vi "MFLMonitor.vi"(0 "Lock-in Reference":u16(ring) items=["Lock-in 1", "Lock-in 2", "Lock-in 3"]) -> ()   [LabVIEW 2019]
uses:
  Utility/Monitor Communication/zurich_lock_in/MFLIMonitor_Cluster.ctl
  Equipment/Zurich Instruments LabOne/Public/Data/ziTypeDemodSampleEx.ctl
  Utility/Monitor Communication/zurich_lock_in/MFLIMonitor-Settings-Cluster.ctl
  Global/Global Variables/Data_Display_global.vi
  Instrument_Setup.vi
  Equipment/Zurich Instruments LabOne/Public/Configure/ziGetValueDouble.vi
  Equipment/Zurich Instruments LabOne/Public/Data/ziGetEventDoubleDataTS.vi
  Equipment/Zurich Instruments LabOne/Public/Data/ziGetEventIntDataTS.vi
  Equipment/Zurich Instruments LabOne/Public/Data/ziGetEventDemodSample.vi
  Equipment/Zurich Instruments LabOne/Public/Configure/ziSetValueDouble.vi
  Equipment/Zurich Instruments LabOne/Zurich Instruments LabOne.lvlib
panel:
  out "Value in Queue":bool
  out "MFLI-1-Settings":T1={"Adress"="DEV4756", "Osc 0 Freq"=0.0, "Osc 1 Freq"=0.0, "Osc 2 Freq"=0.0, "Osc 3 Freq"=0.0, "Demod 0 Osc"=0, "Demod 0 Harm"=1, "Demod 0 Phase"=0.0, "Demod 1 Osc"=0, "Demod 2 Osc"=0, "Demod 3 Osc"=0, "Demod 1 Harm"=1, "Demod 2 Harm"=1, "Demod 3 Harm"=1, "Demod 1 Phase"=0.0, "Demod 2 Phase"=0.0, "Demod 3 Phase"=0.0, "Input Demod 0"="", "Input Demod 1"="", "Input Demod 2"="", "Input Demod 3"="", "Demod 0 Order"=1, "Demod 0 TC"=0.0, "Demod 0 Sinc"=FALSE, "Demod 1 Order"=1, "Demod 2 Order"=1, "Demod 3 Order"=1, "Demod 1 TC"=0.0, "Demod 2 TC"=0.0, "Demod 3 TC"=0.0, "Demod 1 Sinc"=FALSE, "Demod 2 Sinc"=FALSE, "Demod 3 Sinc"=FALSE, "Demod 0 Enable"=FALSE, "Demod 0 Data Rate"=0.0, "Demod 1 Enable"=FALSE, "Demod 2 Enable"=FALSE, "Demod 3 Enable"=FALSE, "Demod 1 Data Rate"=0.0, "Demod 2 Data Rate"=0.0, "Demod 3 Data Rate"=0.0, "Ampl 0"=0.0, "Ampl 0 Enable"=FALSE, "Ampl 1"=0.0, "Ampl 2"=0.0, "Ampl 3"=0.0, "Ampl 1 Enable"=FALSE, "Ampl 2 Enable"=FALSE, "Ampl 3 Enable"=FALSE, "On"=FALSE, "50 Ohm"=FALSE, "Range (V)"=0.0, "Add"=FALSE, "Diff"=FALSE, "Auto-Range"=FALSE, "Offset (V)"=0.0, "Aux Out 0 Select"="", "Aux Out 0 Demod Num"=0.0, "Aux Out 0 Pre Offset"=0.0, "Aux Out 0 Scale"=0.0, "Aux Out 0 Offset"=0.0, "Aux Out 1 Select"="", "Aux Out 2 Select"="", "Aux Out 3 Select"="", "Aux Out 1 Pre Offset"=0.0, "Aux Out 2 Pre Offset"=0.0, "Aux Out 3 Pre Offset"=0.0, "Aux Out 1 Scale"=0.0, "Aux Out 2 Scale"=0.0, "Aux Out 3 Scale"=0.0, "Aux Out 1 Offset"=0.0, "Aux Out 2 Offset"=0.0, "Aux Out 3 Offset"=0.0, "Aux Out 1 Demod Num"=0.0, "Aux Out 2 Demod Num "=0.0, "Aux Out 3 Demod Num"=0.0} {"Aux Out 3 Demod Num" min=0.0 max=3.0 step=1.0; "Aux Out 2 Demod Num" min=0.0 max=3.0 step=1.0; "Aux Out 1 Demod Num" min=0.0 max=3.0 step=1.0; "Aux Out 0 Demod Num" min=0.0 max=3.0 step=1.0; "Demod 3 TC" min=0.0; "Demod 2 TC" min=0.0; "Demod 1 TC" min=0.0; "Demod 3 Order" min=1 max=8 step=1; "Demod 2 Order" min=1 max=8 step=1; "Demod 1 Order" min=1 max=8 step=1; "Demod 0 TC" min=0.0; "Demod 0 Order" min=1 max=8 step=1; "Demod 3 Phase" min=0.0 max=360.0; "Demod 2 Phase" min=0.0 max=360.0; "Demod 1 Phase" min=0.0 max=360.0; "Demod 3 Harm" min=1 max=1023 step=1; "Demod 2 Harm" min=1 max=1023 step=1; "Demod 1 Harm" min=1 max=1023 step=1; "Demod 3 Osc" min=0 max=3 step=1; "Demod 2 Osc" min=0 max=3 step=1; "Demod 1 Osc" min=0 max=3 step=1; "Demod 0 Phase" min=0.0 max=360.0; "Demod 0 Harm" min=1 max=1023 step=1; "Demod 0 Osc" min=0 max=3 step=1; "Osc 3 Freq" min=0.0 max=510000.0 format="%#_11g"; "Osc 2 Freq" min=0.0 max=510000.0 format="%#_11g"; "Osc 1 Freq" min=0.0 max=510000.0 format="%#_11g"; "Osc 0 Freq" min=0.0 max=510000.0 format="%#_11g"}
  in  "Stop":bool
  in  "MFL_Monitor":T2 {"Osc 3 Freq" min=0.0 max=510000.0 format="%#_11g"; "Osc 2 Freq" min=0.0 max=510000.0 format="%#_11g"; "Osc 1 Freq" min=0.0 max=510000.0 format="%#_11g"; "Osc 0 Freq" min=0.0 max=510000.0 format="%#_11g"; "Demod Sample out 3"."Aux In 1 (V)" format="%#_5p"; "Demod Sample out 3"."Aux In 0 (V)" format="%#_5p"; "Demod Sample out 3"."X (Vrms)" format="%#_5p"; "Demod Sample out 3"."Y (Vrms)" format="%#_5p"; "Demod Sample out 3"."Osc Phase (rad)" format="%#.3g"; "Demod Sample out 2"."Aux In 1 (V)" format="%#_5p"; "Demod Sample out 2"."Aux In 0 (V)" format="%#_5p"; "Demod Sample out 2"."X (Vrms)" format="%#_5p"; "Demod Sample out 2"."Y (Vrms)" format="%#_5p"; "Demod Sample out 2"."Osc Phase (rad)" format="%#.3g"; "Demod Sample out 1"."Aux In 1 (V)" format="%#_5p"; "Demod Sample out 1"."Aux In 0 (V)" format="%#_5p"; "Demod Sample out 1"."X (Vrms)" format="%#_5p"; "Demod Sample out 1"."Y (Vrms)" format="%#_5p"; "Demod Sample out 1"."Osc Phase (rad)" format="%#.3g"; "Demod Sample out 0"."Aux In 1 (V)" format="%#_5p"; "Demod Sample out 0"."Aux In 0 (V)" format="%#_5p"; "Demod Sample out 0"."X (Vrms)" format="%#_5p"; "Demod Sample out 0"."Y (Vrms)" format="%#_5p"; "Demod Sample out 0"."Osc Phase (rad)" format="%#.3g"}
  # "Oscillators"
  # "Demodulators"
  # "Low-Pass Filter"
  # "Data Transfer"
  # "Output Amplitudes"
  # "Signal Outputs"
  # "Frequency (Hz)"
  # "Osc (#)"
  # "Harm (#)"
  # "Phase Offset (°)"
  # "Input"
  # "Order (#)"
  # "TC (s)"
  # "Sinc"
  # "Enabled"
  # "Rate (1/s)"
  # "Ampl (Vpk)"
  # "Enable"
  # "0"
  # "0"
  # "0"
  # "1"
  # "1"
  # "1"
  # "2"
  # "2"
  # "2"
  # "3"
  # "3"
  # "3"
  # "Auxiliary Outputs"
  # "Output"
  # "Demod"
  # "Pre Offset"
  # "Scale"
  # "Offset"
  # "0"
  # "1"
  # "2"
  # "3"
  # "Oscillators"
  # "Output Amplitudes"
  # "Frequency (Hz)"
  # "Ampl (Vpk)"
  # "0"
  # "0"
  # "1"
  # "1"
  # "2"
  # "2"
  # "3"
  # "3"
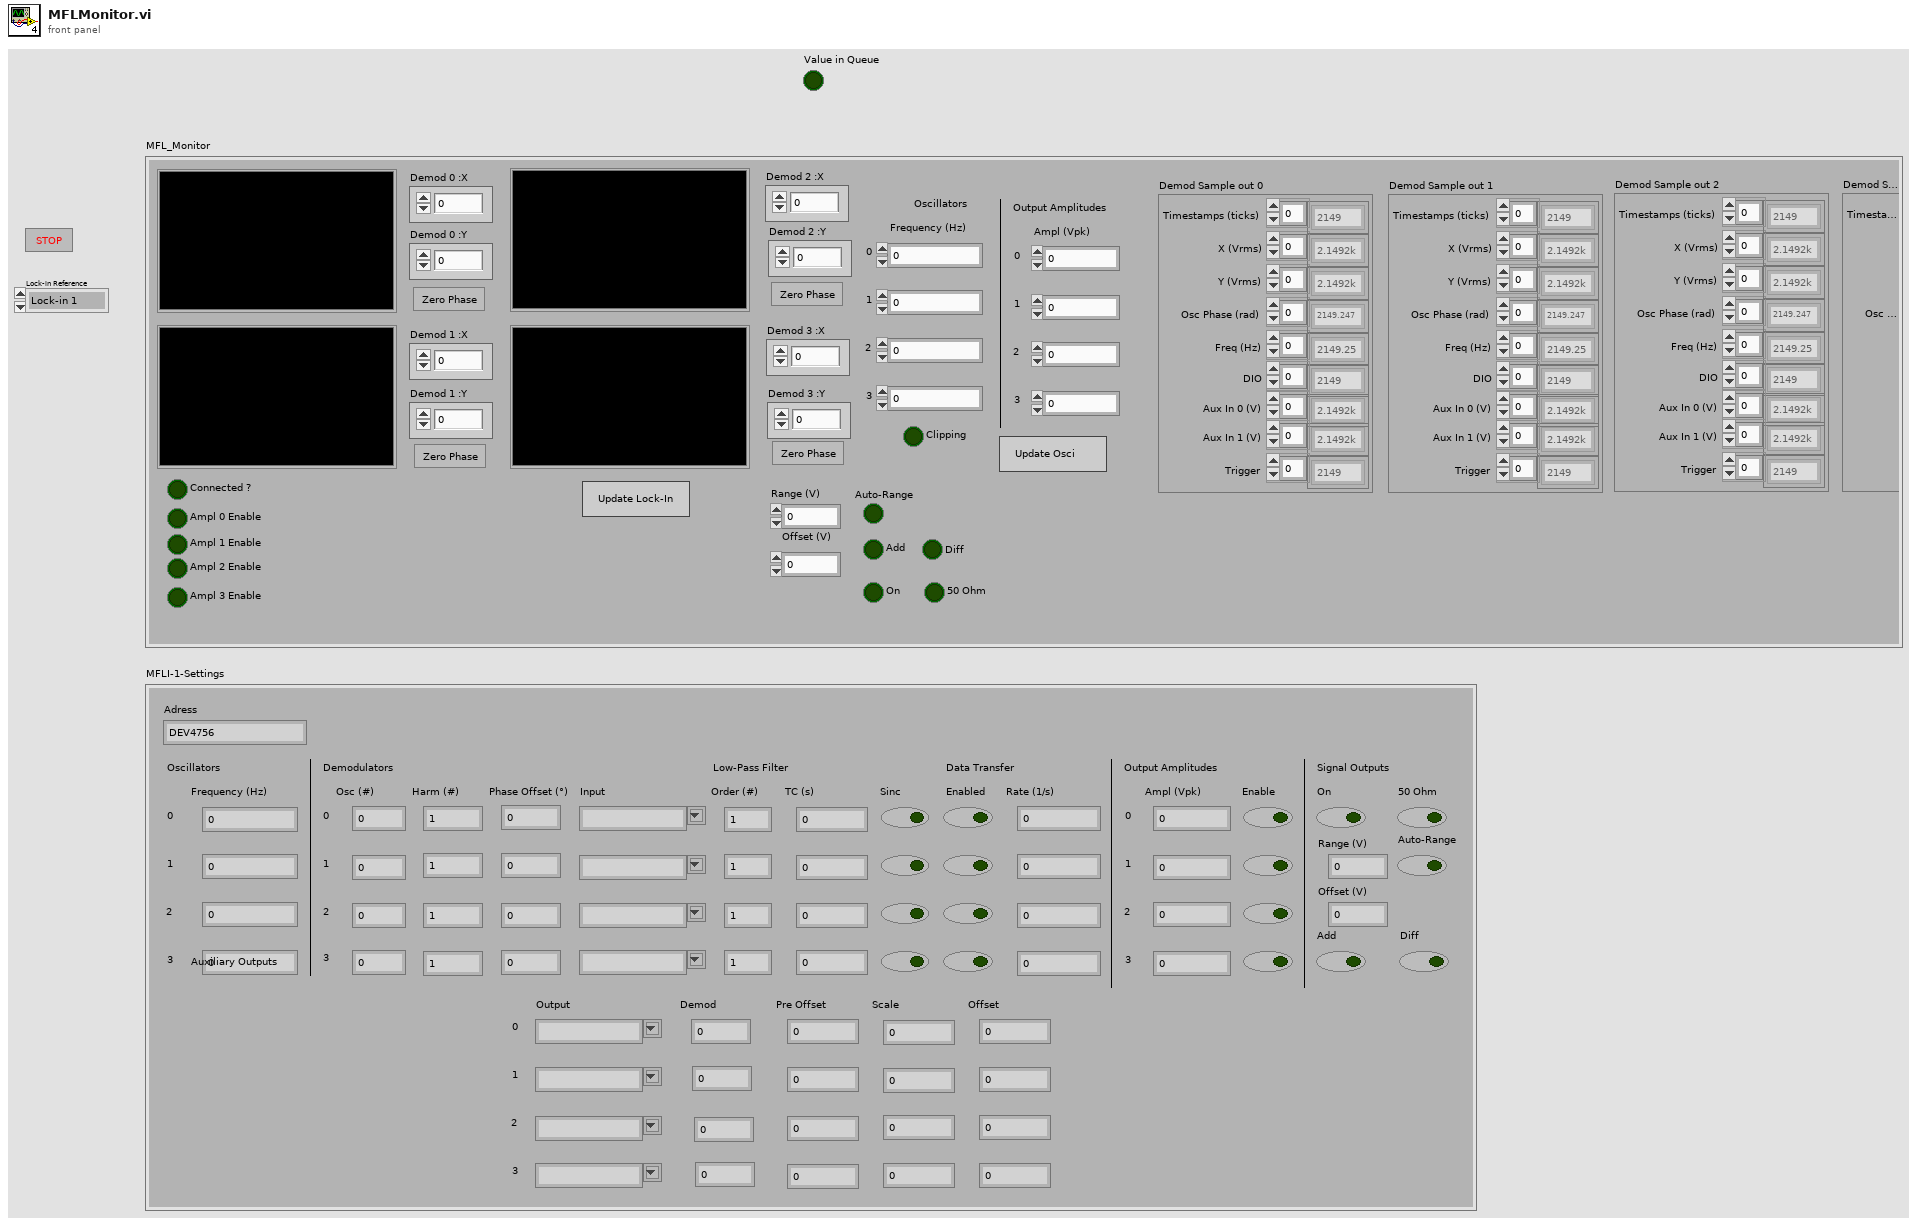
[diagram p1: front panel]
types:
  T1 = typedef "MFLIMonitor-Settings-Cluster.ctl" = cluster{"Adress":string, "Osc 0 Freq":dbl, "Osc 1 Freq":dbl, "Osc 2 Freq":dbl, "Osc 3 Freq":dbl, "Demod 0 Osc":i8, "Demod 0 Harm":i16, "Demod 0 Phase":dbl, "Demod 1 Osc":i8, "Demod 2 Osc":i8, "Demod 3 Osc":i8, "Demod 1 Harm":i16, "Demod 2 Harm":i16, "Demod 3 Harm":i16, "Demod 1 Phase":dbl, "Demod 2 Phase":dbl, "Demod 3 Phase":dbl, "Input Demod 0":string, "Input Demod 1":string, "Input Demod 2":string, "Input Demod 3":string, "Demod 0 Order":i8, "Demod 0 TC":dbl, "Demod 0 Sinc":bool, "Demod 1 Order":i8, "Demod 2 Order":i8, "Demod 3 Order":i8, "Demod 1 TC":dbl, "Demod 2 TC":dbl, "Demod 3 TC":dbl, "Demod 1 Sinc":bool, "Demod 2 Sinc":bool, "Demod 3 Sinc":bool, "Demod 0 Enable":bool, "Demod 0 Data Rate":dbl, "Demod 1 Enable":bool, "Demod 2 Enable":bool, "Demod 3 Enable":bool, "Demod 1 Data Rate":dbl, "Demod 2 Data Rate":dbl, "Demod 3 Data Rate":dbl, "Ampl 0":dbl, "Ampl 0 Enable":bool, "Ampl 1":dbl, "Ampl 2":dbl, "Ampl 3":dbl, "Ampl 1 Enable":bool, "Ampl 2 Enable":bool, "Ampl 3 Enable":bool, "On":bool, "50 Ohm":bool, "Range (V)":dbl, "Add":bool, "Diff":bool, "Auto-Range":bool, "Offset (V)":dbl, "Aux Out 0 Select":string, "Aux Out 0 Demod Num":dbl, "Aux Out 0 Pre Offset":dbl, "Aux Out 0 Scale":dbl, "Aux Out 0 Offset":dbl, "Aux Out 1 Select":string, "Aux Out 2 Select":string, "Aux Out 3 Select":string, "Aux Out 1 Pre Offset":dbl, "Aux Out 2 Pre Offset":dbl, "Aux Out 3 Pre Offset":dbl, "Aux Out 1 Scale":dbl, "Aux Out 2 Scale":dbl, "Aux Out 3 Scale":dbl, "Aux Out 1 Offset":dbl, "Aux Out 2 Offset":dbl, "Aux Out 3 Offset":dbl, "Aux Out 1 Demod Num":dbl, "Aux Out 2 Demod Num ":dbl, "Aux Out 3 Demod Num":dbl}
  T2 = typedef "MFLIMonitor_Cluster.ctl" = cluster{"Demod 0":dbl[][], " Demod 1":dbl[][], "Demod 0 :X":dbl, "Demod 0 :Y ":dbl, "Demod 1 :X":dbl, "Demod 1 :Y ":dbl, " Demod 2":dbl[][], "Demod 3":dbl[][], "Demod 2 :X":dbl, "Demod 2 :Y ":dbl, "Demod 3 :X ":dbl, "Demod 3 :Y ":dbl, "Demod Sample out 0 ":T3, "Demod Sample out 1":T3, "Demod Sample out 2":T3, "Demod Sample out 3":T3, "Update Lock-In":bool, "Connected ?":bool, "Demod 0 Zero Phase":bool, "Demod 1 Zero Phase":bool, "Demod 2 Zero Phase":bool, "Demod 3 Zero Phase":bool, "Osc 0 Freq":dbl, "Osc 1 Freq":dbl, "Osc 2 Freq":dbl, "Osc 3 Freq":dbl, "Clipping":bool, "Range (V)":dbl, "Offset (V)":dbl, "Auto-Range":bool, "Add":bool, "Diff":bool, "On":bool, "50 Ohm":bool, "Ampl 0 Enable":bool, "Ampl 1 Enable":bool, "Ampl 2 Enable":bool, "Ampl 3 Enable":bool, "Ampl 0":dbl, "Ampl 1":dbl, "Ampl 2":dbl, "Ampl 3":dbl, "Update Osci":bool}
  T3 = typedef "Zurich Instruments LabOne.lvlib/ziTypeDemodSampleEx.ctl" = cluster{"Timestamps (ticks)":u64[], "X (Vrms)":dbl[], "Y (Vrms)":dbl[], "Osc Phase (rad)":dbl[], "Freq (Hz)":dbl[], "DIO":u32[], "Aux In 0 (V)":dbl[], "Aux In 1 (V)":dbl[], "Trigger":u32[]}
  T4 = typedef "Zurich Instruments LabOne.lvlib/ziTypeHandle.ctl" = cluster{"handleValid":bool, "Conn":u64, "Path Prefix":string, "Handle":u64, "Connected":bool, "Clockbase(s)":dbl}
  T5 = typedef "Zurich Instruments LabOne.lvlib/ziTypeDoubleDataTS.ctl" = cluster{"Timestamp (ticks)":u64[], "Value":dbl[]}
  T6 = typedef "Zurich Instruments LabOne.lvlib/ziTypeIntegerDataTS.ctl" = cluster{"Timestamp (ticks)":u64[], "Value":i64[]}
  T7 = cluster{"Adress":bool, "Osc 0 Freq":bool, "Osc 1 Freq":bool, "Osc 2 Freq":bool, "Osc 3 Freq":bool, "Demod 0 Osc":bool, "Demod 0 Harm":bool, "Demod 0 Phase":bool, "Demod 1 Osc":bool, "Demod 2 Osc":bool, "Demod 3 Osc":bool, "Demod 1 Harm":bool, "Demod 2 Harm":bool, "Demod 3 Harm":bool, "Demod 1 Phase":bool, "Demod 2 Phase":bool, "Demod 3 Phase":bool, "Input Demod 0":bool, "Input Demod 1":bool, "Input Demod 2":bool, "Input Demod 3":bool, "Demod 0 Order":bool, "Demod 0 TC":bool, "Demod 0 Sinc":bool, "Demod 1 Order":bool, "Demod 2 Order":bool, "Demod 3 Order":bool, "Demod 1 TC":bool, "Demod 2 TC":bool, "Demod 3 TC":bool, "Demod 1 Sinc":bool, "Demod 2 Sinc":bool, "Demod 3 Sinc":bool, "Demod 0 Enable":bool, "Demod 0 Data Rate":bool, "Demod 1 Enable":bool, "Demod 2 Enable":bool, "Demod 3 Enable":bool, "Demod 1 Data Rate":bool, "Demod 2 Data Rate":bool, "Demod 3 Data Rate":bool, "Ampl 0":bool, "Ampl 0 Enable":bool, "Ampl 1":bool, "Ampl 2":bool, "Ampl 3":bool, "Ampl 1 Enable":bool, "Ampl 2 Enable":bool, "Ampl 3 Enable":bool, "On":bool, "50 Ohm":bool, "Range (V)":bool, "Add":bool, "Diff":bool, "Auto-Range":bool, "Offset (V)":bool, "Aux Out 0 Select":bool, "Aux Out 0 Demod Num":bool, "Aux Out 0 Pre Offset":bool, "Aux Out 0 Scale":bool, "Aux Out 0 Offset":bool, "Aux Out 1 Select":bool, "Aux Out 2 Select":bool, "Aux Out 3 Select":bool, "Aux Out 1 Pre Offset":bool, "Aux Out 2 Pre Offset":bool, "Aux Out 3 Pre Offset":bool, "Aux Out 1 Scale":bool, "Aux Out 2 Scale":bool, "Aux Out 3 Scale":bool, "Aux Out 1 Offset":bool, "Aux Out 2 Offset":bool, "Aux Out 3 Offset":bool, "Aux Out 1 Demod Num":bool, "Aux Out 2 Demod Num ":bool, "Aux Out 3 Demod Num":bool}
  T8 = cluster{"Sensitivity Setpoint 1":i32, "Sensitivity Setpoint 2":i32, "Sensitivity Setpoint 3":i32}
  T9 = cluster{"LIA7230-Running":bool, "LIA7230-Running 2":bool, "LIA7230-Running 3":bool, "SR830-Running":bool, "SR830-Running 2":bool, "SR830-Running 3":bool, "PE7265-running":bool, "zurich_Lock_in-running":bool}
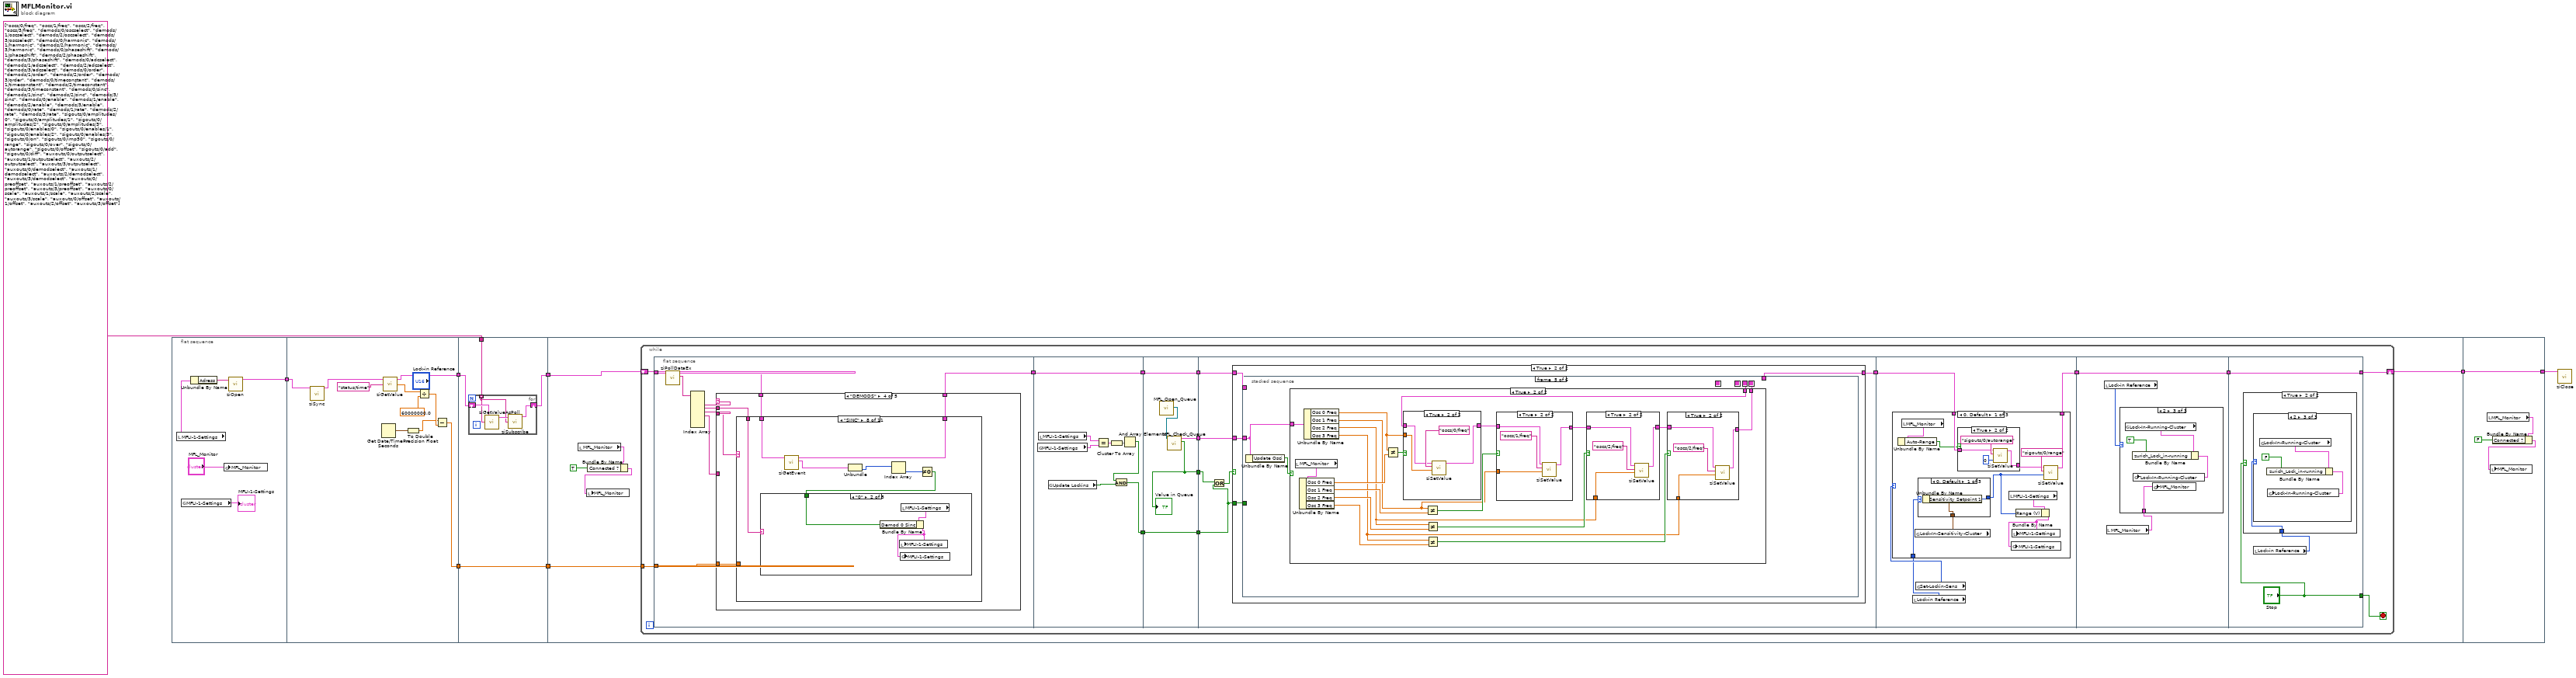
[diagram p0: block diagram]
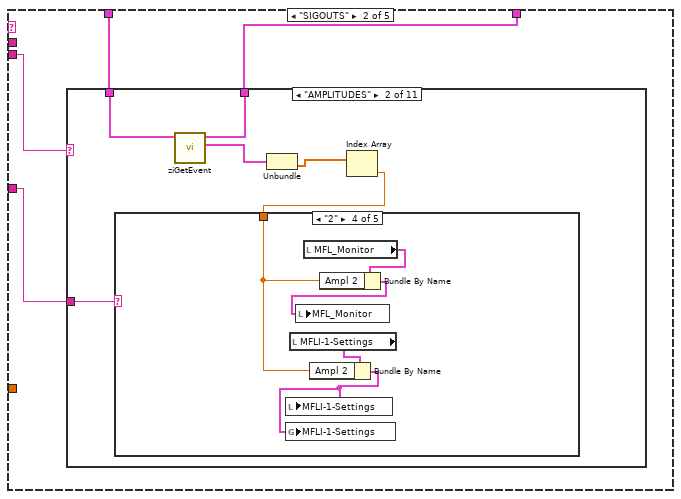
[diagram p3: hidden frame]
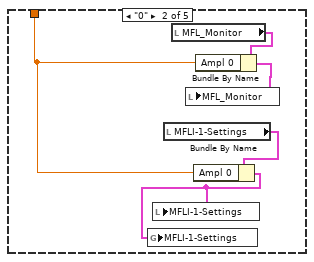
[diagram p6: hidden frame]
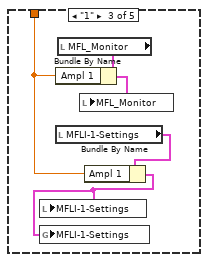
[diagram p7: hidden frame]
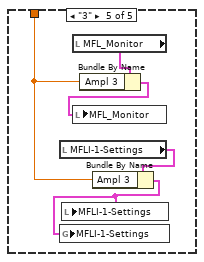
[diagram p8: hidden frame]
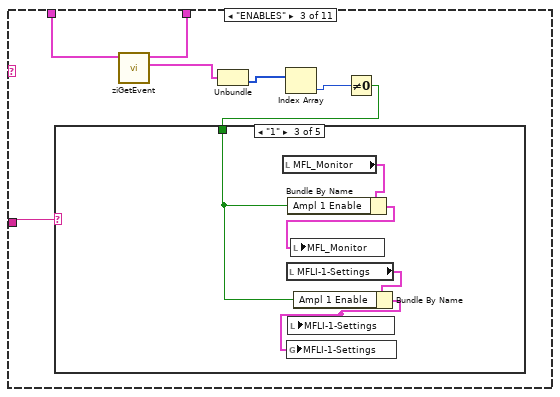
[diagram p9: hidden frame]
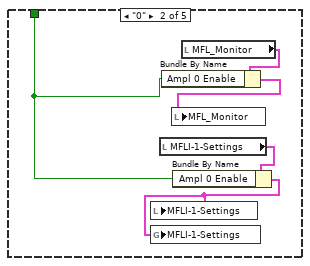
[diagram p11: hidden frame]
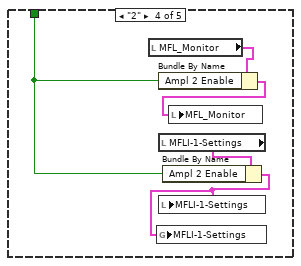
[diagram p12: hidden frame]
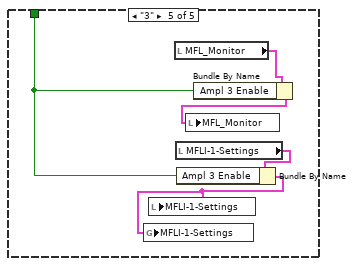
[diagram p13: hidden frame]
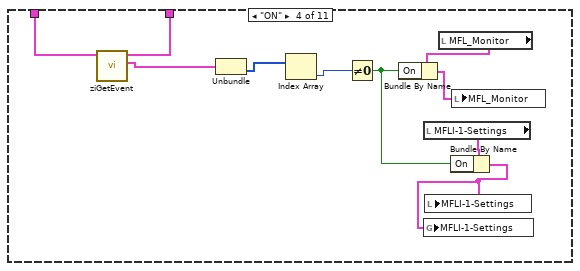
[diagram p14: hidden frame]
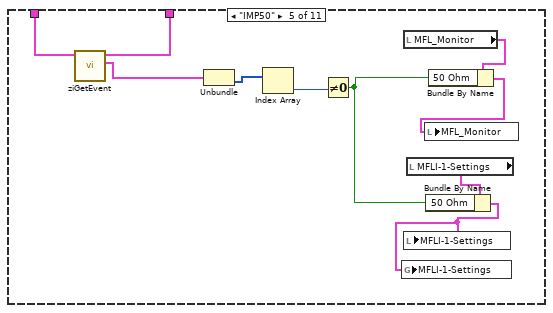
[diagram p15: hidden frame]
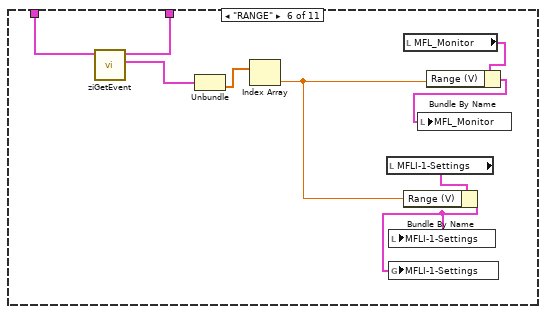
[diagram p16: hidden frame]
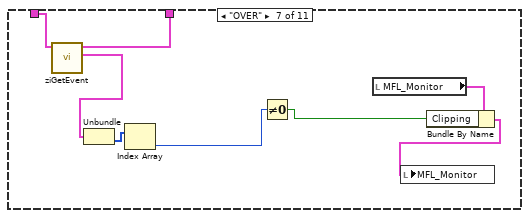
[diagram p17: hidden frame]
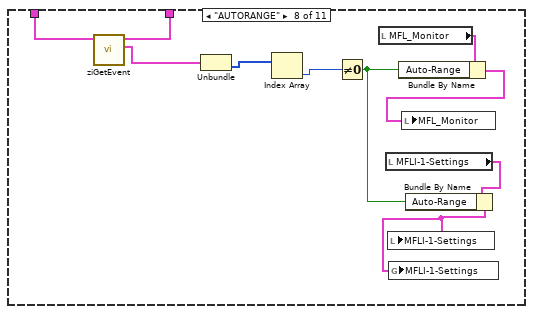
[diagram p18: hidden frame]
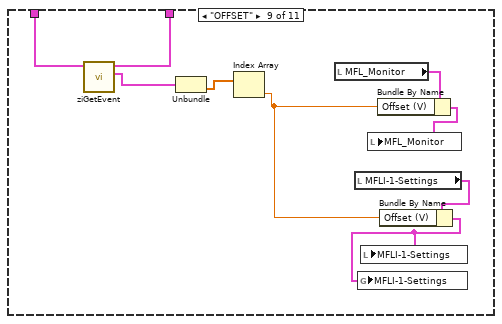
[diagram p19: hidden frame]
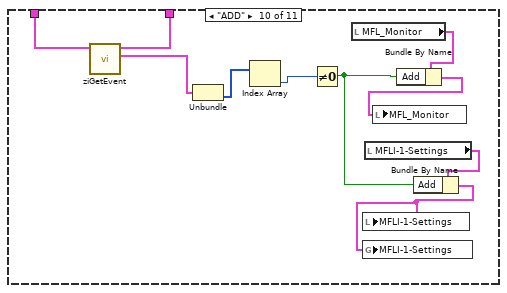
[diagram p20: hidden frame]
diagram:
  n1 = flat-sequence {
    tunnel: [w13] -> w7
    tunnel: [w17] -> w6
    tunnel: w7 -> [w15]
    tunnel: [w16] -> w5
    tunnel: w6 -> [w27]
    tunnel: w5 -> [w26]
    tunnel: [w26] -> w4
    tunnel: string[] ["oscs/0/freq", "oscs/1/freq", "oscs/2/freq", "oscs/3/freq", "demods/0/oscselect", "demods/1/oscselect", "demods/2/oscselect", "demods/3/oscselect", "demods/0/harmonic", "demods/1/harmonic", "demods/2/harmonic", "demods/3/harmonic", "demods/0/phaseshift", "demods/1/phaseshift", "demods/2/phaseshift", "demods/3/phaseshift", "demods/0/adcselect", "demods/1/adcselect", "demods/2/adcselect", "demods/3/adcselect", "demods/0/order", "demods/1/order", "demods/2/order", "demods/3/order", "demods/0/timeconstant", "demods/1/timeconstant", "demods/2/timeconstant", "demods/3/timeconstant", "demods/0/sinc", "demods/1/sinc", "demods/2/sinc", "demods/3/sinc", "demods/0/enable", "demods/1/enable", "demods/2/enable", "demods/3/enable", "demods/0/rate", "demods/1/rate", "demods/2/rate", "demods/3/rate", "sigouts/0/amplitudes/0", "sigouts/0/amplitudes/1", "sigouts/0/amplitudes/2", "sigouts/0/amplitudes/3", "sigouts/0/enables/0", "sigouts/0/enables/1", "sigouts/0/enables/2", "sigouts/0/enables/3", "sigouts/0/on", "sigouts/0/imp50", "sigouts/0/range", "sigouts/0/over", "sigouts/0/autorange", "sigouts/0/offset", "sigouts/0/add", "sigouts/0/diff", "auxouts/0/outputselect", "auxouts/1/outputselect", "auxouts/2/outputselect", "auxouts/3/outputselect", "auxouts/0/demodselect", "auxouts/1/demodselect", "auxouts/2/demodselect", "auxouts/3/demodselect", "auxouts/0/preoffset", "auxouts/1/preoffset", "auxouts/2/preoffset", "auxouts/3/preoffset", "auxouts/0/scale", "auxouts/1/scale", "auxouts/2/scale", "auxouts/3/scale", "auxouts/0/offset", "auxouts/1/offset", "auxouts/2/offset", "auxouts/3/offset"] -> [w25]
    tunnel: [w24] -> w2
    tunnel: w4 -> [w36]
    tunnel: w2 -> [w35]
    tunnel: [w37] -> w1
    tunnel: [w1246] -> w8
    tunnel: w1 -> [w1246]
    frame #0 {
      n2 = local read "MFLI-1-Settings"() -> (w12:T1)
      n3 = global read "Instrument_Setup.vi" "MFLI-1-Settings"() -> (→"MFLI-1-Settings":T1)
      n4 = Unbundle By Name(w12) -> ("Adress"=w11:string)
      n5 = global write "Data_Display_global.vi" "MFL_Monitor"("MFL_Monitor") -> ()
      n6 = call "ziOpen.vi"("Address"=w11) -> ("HandleOut"=w13:T4)  [unwired: 3 in, 2 out]
    }
    frame #1 {
      n7 = call "ziSync.vi"("Handle In"=w15) -> ("Handle Out"=w14:T4)  [unwired: 13 in, 1 out]
      n8 = Get Date/Time In Seconds() -> (seconds since 1Jan1904=w19:timestamp)
      n9 = call-poly "ziGetValue.vi"("Path"="status/time", "Handle in"=w14) -> ("Value"=w22:dbl, "Handle out"=w17:T4)  [unwired: 1 in, 1 out]
      n10 = To Double Precision Float(number=w19) -> (double precision float=w18:dbl)
      n11 = Divide(x=w22, y=60000000.0) -> (x/y=w20:dbl)
      n12 = Subtract(x=w18, y=w20) -> (x-y=w16:dbl)
    }
    frame #2 {
      n13 = for {
        shift-right: [w29] -> w24
        shift-left: w27 -> [w31]
        tunnel: w25 -> [w28] mode=indexing
        n14 = call "ziGetValueAsPoll.vi"("Path"=w28, "Handle in"=w31) -> ("Handle out"=w30:T4)  [unwired: 2 in, 1 out]
        n15 = call "ziSubscribe.vi"("Path ()"=w28, "Handle In"=w30) -> ("Handle Out"=w29:T4)  [unwired: 2 in, 1 out]
      }
    }
    frame #3 {
      n16 = local read "MFL_Monitor"() -> (w34:T2)
      n17 = Bundle By Name(cluster=w34, "Connected ?"=TRUE) -> (w33:T2)
      n18 = local write "MFL_Monitor"(w33) -> ()
      n19 = while {
        shift-right: [w50] -> w37
        shift-left: w35 -> [w51]
        tunnel: w36 -> [w49]
        stop <- w47 stop-if-true
        n20 = flat-sequence {
          tunnel: [w53] -> w41
          tunnel: w49 -> [w52]
          tunnel: w51 -> [w60]
          tunnel: w41 -> [w589]
          tunnel: [w589] -> w40
          tunnel: [w582] -> w39
          tunnel: w40 -> [w594]
          tunnel: [w594] -> w48
          tunnel: [w591] -> w45
          tunnel: [w592] -> w44
          tunnel: w39 -> [w590]
          tunnel: [w590] -> w38
          tunnel: [w599] -> w43
          tunnel: w48 -> [w600]
          tunnel: w45 -> [w597]
          tunnel: w44 -> [w598]
          tunnel: w38 -> [w595]
          tunnel: w43 -> [w1173]
          tunnel: [w1172] -> w42
          tunnel: [w1217] -> w46
          tunnel: w42 -> [w1217]
          tunnel: ["Stop"] -> w47
          tunnel: [w1232] -> w50
          tunnel: w46 -> [w1232]
          frame #0 {
            n21 = call "ziPollDataEx.vi"("Handle In"=w60) -> ("PathArray"=w59:string[], "Handle Out"=w57:T4)  [unwired: 3 in, 6 out]
            n22 = Index Array(array=w59) -> (element #2=w58:string, element #3=w55:string, element #4=w56:string, element #5=w54:string)  [unwired: 8 in, 4 out]
            n23 = case shown="\"DEMODS\"" w58 {
              tunnel: w56 -> [_ w65 w198 w229 w489]
              tunnel: w57 -> [w61 w64 w202 w227 w487]
              tunnel: w55 -> [_ _ w197 w228 w488]
              tunnel: w54 -> [_ w63 _ _ _]
              tunnel: [w61 w62 w196 w226 w486] -> w53
              tunnel: w52 -> [_ _ _ w225 _]
              frame Default {
              }
              frame "SIGOUTS" {
                n24 = case shown="\"AMPLITUDES\"" w65 {
                  tunnel: w64 -> [w66 w72 w99 w129 w139 w148 w156 w166 w175 w185 w195]
                  tunnel: [w66 w71 w98 w128 w138 w147 w155 w165 w174 w184 w194] -> w62
                  tunnel: w63 -> [_ w67 w93 _ _ _ _ _ _ _ _]
                  frame Default {
                  }
                  frame "AMPLITUDES" {
                    n25 = call-poly "ziGetEvent.vi"("Handle In"=w72) -> ("Sample Out"=w70:T5, "Handle Out"=w71:T4)  [unwired: 8 in, 1 out]
                    n26 = Unbundle(w70) -> ("Value"=w69:dbl[])  [unwired: 1 out]
                    n27 = Index Array(array=w69) -> (element=w68:dbl)  [unwired: 1 in]
                    n28 = case shown="\"2\"" w67 {
                      tunnel: w68 -> [_ w74 w79 w84 w89]
                      frame Default {
                      }
                      frame "0" {
                        n29 = local read "MFLI-1-Settings"() -> (w75:T1)
                        n30 = local read "MFL_Monitor"() -> (w77:T2)
                        n31 = Bundle By Name(cluster=w75, "Ampl 0"=w74) -> (w73:T1)
                        n32 = global write "Instrument_Setup.vi" "MFLI-1-Settings"(w73) -> ()
                        n33 = local write "MFLI-1-Settings"(w73) -> ()
                        n34 = Bundle By Name(cluster=w77, "Ampl 0"=w74) -> (w76:T2)
                        n35 = local write "MFL_Monitor"(w76) -> ()
                      }
                      frame "1" {
                        n36 = local read "MFLI-1-Settings"() -> (w80:T1)
                        n37 = local read "MFL_Monitor"() -> (w82:T2)
                        n38 = Bundle By Name(cluster=w82, "Ampl 1"=w79) -> (w81:T2)
                        n39 = local write "MFL_Monitor"(w81) -> ()
                        n40 = Bundle By Name(cluster=w80, "Ampl 1"=w79) -> (w78:T1)
                        n41 = local write "MFLI-1-Settings"(w78) -> ()
                        n42 = global write "Instrument_Setup.vi" "MFLI-1-Settings"(w78) -> ()
                      }
                      frame "2" {
                        n43 = local read "MFLI-1-Settings"() -> (w85:T1)
                        n44 = local read "MFL_Monitor"() -> (w87:T2)
                        n45 = Bundle By Name(cluster=w85, "Ampl 2"=w84) -> (w83:T1)
                        n46 = local write "MFLI-1-Settings"(w83) -> ()
                        n47 = global write "Instrument_Setup.vi" "MFLI-1-Settings"(w83) -> ()
                        n48 = Bundle By Name(cluster=w87, "Ampl 2"=w84) -> (w86:T2)
                        n49 = local write "MFL_Monitor"(w86) -> ()
                      }
                      frame "3" {
                        n50 = local read "MFLI-1-Settings"() -> (w90:T1)
                        n51 = local read "MFL_Monitor"() -> (w92:T2)
                        n52 = Bundle By Name(cluster=w92, "Ampl 3"=w89) -> (w91:T2)
                        n53 = local write "MFL_Monitor"(w91) -> ()
                        n54 = Bundle By Name(cluster=w90, "Ampl 3"=w89) -> (w88:T1)
                        n55 = global write "Instrument_Setup.vi" "MFLI-1-Settings"(w88) -> ()
                        n56 = local write "MFLI-1-Settings"(w88) -> ()
                      }
                    }
                  }
                  frame "ENABLES" {
                    n57 = call-poly "ziGetEvent.vi"("Handle In"=w99) -> ("Sample Out"=w97:T6, "Handle Out"=w98:T4)  [unwired: 8 in, 1 out]
                    n58 = Unbundle(w97) -> ("Value"=w96:i64[])  [unwired: 1 out]
                    n59 = Index Array(array=w96) -> (element=w95:i64)  [unwired: 1 in]
                    n60 = Not Equal To 0?(x=w95) -> (x != 0?=w94:bool)
                    n61 = case shown="\"1\"" w93 {
                      tunnel: w94 -> [_ w101 w106 w111 w116]
                      frame Default {
                      }
                      frame "0" {
                        n62 = local read "MFLI-1-Settings"() -> (w102:T1)
                        n63 = Bundle By Name(cluster=w102, "Ampl 0 Enable"=w101) -> (w100:T1)
                        n64 = local write "MFLI-1-Settings"(w100) -> ()
                        n65 = global write "Instrument_Setup.vi" "MFLI-1-Settings"(w100) -> ()
                        n66 = local read "MFL_Monitor"() -> (w104:T2)
                        n67 = Bundle By Name(cluster=w104, "Ampl 0 Enable"=w101) -> (w103:T2)
                        n68 = local write "MFL_Monitor"(w103) -> ()
                      }
                      frame "1" {
                        n69 = local read "MFL_Monitor"() -> (w109:T2)
                        n70 = local read "MFLI-1-Settings"() -> (w107:T1)
                        n71 = Bundle By Name(cluster=w109, "Ampl 1 Enable"=w106) -> (w108:T2)
                        n72 = local write "MFL_Monitor"(w108) -> ()
                        n73 = Bundle By Name(cluster=w107, "Ampl 1 Enable"=w106) -> (w105:T1)
                        n74 = global write "Instrument_Setup.vi" "MFLI-1-Settings"(w105) -> ()
                        n75 = local write "MFLI-1-Settings"(w105) -> ()
                      }
                      frame "2" {
                        n76 = local read "MFL_Monitor"() -> (w114:T2)
                        n77 = Bundle By Name(cluster=w114, "Ampl 2 Enable"=w111) -> (w113:T2)
                        n78 = local read "MFLI-1-Settings"() -> (w112:T1)
                        n79 = Bundle By Name(cluster=w112, "Ampl 2 Enable"=w111) -> (w110:T1)
                        n80 = global write "Instrument_Setup.vi" "MFLI-1-Settings"(w110) -> ()
                        n81 = local write "MFLI-1-Settings"(w110) -> ()
                        n82 = local write "MFL_Monitor"(w113) -> ()
                      }
                      frame "3" {
                        n83 = local read "MFL_Monitor"() -> (w119:T2)
                        n84 = local read "MFLI-1-Settings"() -> (w117:T1)
                        n85 = Bundle By Name(cluster=w117, "Ampl 3 Enable"=w116) -> (w115:T1)
                        n86 = global write "Instrument_Setup.vi" "MFLI-1-Settings"(w115) -> ()
                        n87 = local write "MFLI-1-Settings"(w115) -> ()
                        n88 = Bundle By Name(cluster=w119, "Ampl 3 Enable"=w116) -> (w118:T2)
                        n89 = local write "MFL_Monitor"(w118) -> ()
                      }
                    }
                  }
                  frame "ON" {
                    n90 = call-poly "ziGetEvent.vi"("Handle In"=w129) -> ("Sample Out"=w127:T6, "Handle Out"=w128:T4)  [unwired: 8 in, 1 out]
                    n91 = Unbundle(w127) -> ("Value"=w126:i64[])  [unwired: 1 out]
                    n92 = Index Array(array=w126) -> (element=w125:i64)  [unwired: 1 in]
                    n93 = Not Equal To 0?(x=w125) -> (x != 0?=w121:bool)
                    n94 = local read "MFLI-1-Settings"() -> (w122:T1)
                    n95 = local read "MFL_Monitor"() -> (w124:T2)
                    n96 = Bundle By Name(cluster=w124, "On"=w121) -> (w123:T2)
                    n97 = Bundle By Name(cluster=w122, "On"=w121) -> (w120:T1)
                    n98 = global write "Instrument_Setup.vi" "MFLI-1-Settings"(w120) -> ()
                    n99 = local write "MFLI-1-Settings"(w120) -> ()
                    n100 = local write "MFL_Monitor"(w123) -> ()
                  }
                  frame "IMP50" {
                    n101 = call-poly "ziGetEvent.vi"("Handle In"=w139) -> ("Sample Out"=w137:T6, "Handle Out"=w138:T4)  [unwired: 8 in, 1 out]
                    n102 = Unbundle(w137) -> ("Value"=w136:i64[])  [unwired: 1 out]
                    n103 = Index Array(array=w136) -> (element=w135:i64)  [unwired: 1 in]
                    n104 = Not Equal To 0?(x=w135) -> (x != 0?=w131:bool)
                    n105 = local read "MFL_Monitor"() -> (w134:T2)
                    n106 = local read "MFLI-1-Settings"() -> (w132:T1)
                    n107 = Bundle By Name(cluster=w132, "50 Ohm"=w131) -> (w130:T1)
                    n108 = global write "Instrument_Setup.vi" "MFLI-1-Settings"(w130) -> ()
                    n109 = local write "MFLI-1-Settings"(w130) -> ()
                    n110 = Bundle By Name(cluster=w134, "50 Ohm"=w131) -> (w133:T2)
                    n111 = local write "MFL_Monitor"(w133) -> ()
                  }
                  frame "RANGE" {
                    n112 = call-poly "ziGetEvent.vi"("Handle In"=w148) -> ("Sample Out"=w146:T5, "Handle Out"=w147:T4)  [unwired: 8 in, 1 out]
                    n113 = Unbundle(w146) -> ("Value"=w145:dbl[])  [unwired: 1 out]
                    n114 = Index Array(array=w145) -> (element=w141:dbl)  [unwired: 1 in]
                    n115 = local read "MFLI-1-Settings"() -> (w142:T1)
                    n116 = local read "MFL_Monitor"() -> (w144:T2)
                    n117 = Bundle By Name(cluster=w142, "Range (V)"=w141) -> (w140:T1)
                    n118 = local write "MFLI-1-Settings"(w140) -> ()
                    n119 = global write "Instrument_Setup.vi" "MFLI-1-Settings"(w140) -> ()
                    n120 = Bundle By Name(cluster=w144, "Range (V)"=w141) -> (w143:T2)
                    n121 = local write "MFL_Monitor"(w143) -> ()
                  }
                  frame "OVER" {
                    n122 = call-poly "ziGetEvent.vi"("Handle In"=w156) -> ("Sample Out"=w154:T6, "Handle Out"=w155:T4)  [unwired: 8 in, 1 out]
                    n123 = Unbundle(w154) -> ("Value"=w153:i64[])  [unwired: 1 out]
                    n124 = Index Array(array=w153) -> (element=w152:i64)  [unwired: 1 in]
                    n125 = Not Equal To 0?(x=w152) -> (x != 0?=w149:bool)
                    n126 = local read "MFL_Monitor"() -> (w151:T2)
                    n127 = Bundle By Name(cluster=w151, "Clipping"=w149) -> (w150:T2)
                    n128 = local write "MFL_Monitor"(w150) -> ()
                  }
                  frame "AUTORANGE" {
                    n129 = call-poly "ziGetEvent.vi"("Handle In"=w166) -> ("Sample Out"=w164:T6, "Handle Out"=w165:T4)  [unwired: 8 in, 1 out]
                    n130 = Unbundle(w164) -> ("Value"=w163:i64[])  [unwired: 1 out]
                    n131 = Index Array(array=w163) -> (element=w162:i64)  [unwired: 1 in]
                    n132 = Not Equal To 0?(x=w162) -> (x != 0?=w158:bool)
                    n133 = local read "MFL_Monitor"() -> (w161:T2)
                    n134 = local read "MFLI-1-Settings"() -> (w159:T1)
                    n135 = Bundle By Name(cluster=w161, "Auto-Range"=w158) -> (w160:T2)
                    n136 = local write "MFL_Monitor"(w160) -> ()
                    n137 = Bundle By Name(cluster=w159, "Auto-Range"=w158) -> (w157:T1)
                    n138 = local write "MFLI-1-Settings"(w157) -> ()
                    n139 = global write "Instrument_Setup.vi" "MFLI-1-Settings"(w157) -> ()
                  }
                  frame "OFFSET" {
                    n140 = call-poly "ziGetEvent.vi"("Handle In"=w175) -> ("Sample Out"=w173:T5, "Handle Out"=w174:T4)  [unwired: 8 in, 1 out]
                    n141 = Unbundle(w173) -> ("Value"=w172:dbl[])  [unwired: 1 out]
                    n142 = Index Array(array=w172) -> (element=w168:dbl)  [unwired: 1 in]
                    n143 = local read "MFL_Monitor"() -> (w171:T2)
                    n144 = local read "MFLI-1-Settings"() -> (w169:T1)
                    n145 = Bundle By Name(cluster=w171, "Offset (V)"=w168) -> (w170:T2)
                    n146 = local write "MFL_Monitor"(w170) -> ()
                    n147 = Bundle By Name(cluster=w169, "Offset (V)"=w168) -> (w167:T1)
                    n148 = global write "Instrument_Setup.vi" "MFLI-1-Settings"(w167) -> ()
                    n149 = local write "MFLI-1-Settings"(w167) -> ()
                  }
                  frame "ADD" {
                    n150 = call-poly "ziGetEvent.vi"("Handle In"=w185) -> ("Sample Out"=w183:T6, "Handle Out"=w184:T4)  [unwired: 8 in, 1 out]
                    n151 = Unbundle(w183) -> ("Value"=w182:i64[])  [unwired: 1 out]
                    n152 = Index Array(array=w182) -> (element=w181:i64)  [unwired: 1 in]
                    n153 = Not Equal To 0?(x=w181) -> (x != 0?=w177:bool)
                    n154 = local read "MFL_Monitor"() -> (w180:T2)
                    n155 = local read "MFLI-1-Settings"() -> (w178:T1)
                    n156 = Bundle By Name(cluster=w180, "Add"=w177) -> (w179:T2)
                    n157 = local write "MFL_Monitor"(w179) -> ()
                    n158 = Bundle By Name(cluster=w178, "Add"=w177) -> (w176:T1)
                    n159 = local write "MFLI-1-Settings"(w176) -> ()
                    n160 = global write "Instrument_Setup.vi" "MFLI-1-Settings"(w176) -> ()
                  }
                  frame "DIFF" {
                    n161 = call-poly "ziGetEvent.vi"("Handle In"=w195) -> ("Sample Out"=w193:T6, "Handle Out"=w194:T4)  [unwired: 8 in, 1 out]
                    n162 = Unbundle(w193) -> ("Value"=w192:i64[])  [unwired: 1 out]
                    n163 = Index Array(array=w192) -> (element=w191:i64)  [unwired: 1 in]
                    n164 = Not Equal To 0?(x=w191) -> (x != 0?=w187:bool)
                    n165 = local read "MFL_Monitor"() -> (w190:T2)
                    n166 = local read "MFLI-1-Settings"() -> (w188:T1)
                    n167 = Bundle By Name(cluster=w190, "Diff"=w187) -> (w189:T2)
                    n168 = local write "MFL_Monitor"(w189) -> ()
                    n169 = Bundle By Name(cluster=w188, "Diff"=w187) -> (w186:T1)
                    n170 = local write "MFLI-1-Settings"(w186) -> ()
                    n171 = global write "Instrument_Setup.vi" "MFLI-1-Settings"(w186) -> ()
                  }
                }
              }
              frame "OSCS" {
                n172 = call-poly "ziGetEvent.vi"("Handle In"=w202) -> ("Sample Out"=w201:T5, "Handle Out"=w196:T4)  [unwired: 8 in, 1 out]
                n173 = Unbundle(w201) -> ("Value"=w200:dbl[])  [unwired: 1 out]
                n174 = Index Array(array=w200) -> (element=w199:dbl)  [unwired: 1 in]
                n175 = case shown="\"FREQ\"" w198 {
                  tunnel: w199 -> [_ w204]
                  tunnel: w197 -> [_ w203]
                  frame Default {
                  }
                  frame "FREQ" {
                    n176 = case shown="Default" w203 {
                      tunnel: w204 -> [_ w206 w211 w216 w221]
                      frame Default {
                      }
                      frame "0" {
                        n177 = local read "MFLI-1-Settings"() -> (w209:T1)
                        n178 = local read "MFL_Monitor"() -> (w208:T2)
                        n179 = Bundle By Name(cluster=w209, "Osc 0 Freq"=w206) -> (w205:T1)
                        n180 = local write "MFLI-1-Settings"(w205) -> ()
                        n181 = global write "Instrument_Setup.vi" "MFLI-1-Settings"(w205) -> ()
                        n182 = Bundle By Name(cluster=w208, "Osc 0 Freq"=w206) -> (w207:T2)
                        n183 = local write "MFL_Monitor"(w207) -> ()
                      }
                      frame "1" {
                        n184 = local read "MFLI-1-Settings"() -> (w214:T1)
                        n185 = local read "MFL_Monitor"() -> (w213:T2)
                        n186 = Bundle By Name(cluster=w213, "Osc 1 Freq"=w211) -> (w212:T2)
                        n187 = local write "MFL_Monitor"(w212) -> ()
                        n188 = Bundle By Name(cluster=w214, "Osc 1 Freq"=w211) -> (w210:T1)
                        n189 = local write "MFLI-1-Settings"(w210) -> ()
                        n190 = global write "Instrument_Setup.vi" "MFLI-1-Settings"(w210) -> ()
                      }
                      frame "2" {
                        n191 = local read "MFLI-1-Settings"() -> (w219:T1)
                        n192 = local read "MFL_Monitor"() -> (w218:T2)
                        n193 = Bundle By Name(cluster=w219, "Osc 2 Freq"=w216) -> (w215:T1)
                        n194 = local write "MFLI-1-Settings"(w215) -> ()
                        n195 = global write "Instrument_Setup.vi" "MFLI-1-Settings"(w215) -> ()
                        n196 = Bundle By Name(cluster=w218, "Osc 2 Freq"=w216) -> (w217:T2)
                        n197 = local write "MFL_Monitor"(w217) -> ()
                      }
                      frame "3" {
                        n198 = local read "MFLI-1-Settings"() -> (w224:T1)
                        n199 = local read "MFL_Monitor"() -> (w223:T2)
                        n200 = Bundle By Name(cluster=w224, "Osc 3 Freq"=w221) -> (w220:T1)
                        n201 = global write "Instrument_Setup.vi" "MFLI-1-Settings"(w220) -> ()
                        n202 = local write "MFLI-1-Settings"(w220) -> ()
                        n203 = Bundle By Name(cluster=w223, "Osc 3 Freq"=w221) -> (w222:T2)
                        n204 = local write "MFL_Monitor"(w222) -> ()
                      }
                    }
                  }
                }
              }
              frame "DEMODS" {
                n205 = case shown="\"SINC\"" w229 {
                  tunnel: w228 -> [_ w235 w250 w271 w287 w311 w327 w347 w364 w421 w444]
                  tunnel: w227 -> [w230 w236 w254 w272 w290 w312 w330 w344 w369 w424 w445]
                  tunnel: [w230 w231 w249 w267 w285 w307 w325 w343 w362 w419 w440] -> w226
                  tunnel: w225 -> [_ _ _ _ _ _ _ _ _ _ w439]
                  frame Default {
                  }
                  frame "OSCSELECT" {
                    n206 = call-poly "ziGetEvent.vi"("Handle In"=w236) -> ("Sample Out"=w234:T6, "Handle Out"=w231:T4)  [unwired: 8 in, 1 out]
                    n207 = Unbundle(w234) -> ("Value"=w233:i64[])  [unwired: 1 out]
                    n208 = Index Array(array=w233) -> (element=w232:i64)  [unwired: 1 in]
                    n209 = case shown="\"3\"" w235 {
                      tunnel: w232 -> [_ w238 w241 w244 w247]
                      frame Default {
                      }
                      frame "0" {
                        n210 = local read "MFLI-1-Settings"() -> (w239:T1)
                        n211 = Bundle By Name(cluster=w239, "Demod 0 Osc"=w238) -> (w237:T1)
                        n212 = global write "Instrument_Setup.vi" "MFLI-1-Settings"(w237) -> ()
                        n213 = local write "MFLI-1-Settings"(w237) -> ()
                      }
                      frame "1" {
                        n214 = local read "MFLI-1-Settings"() -> (w242:T1)
                        n215 = Bundle By Name(cluster=w242, "Demod 1 Osc"=w241) -> (w240:T1)
                        n216 = global write "Instrument_Setup.vi" "MFLI-1-Settings"(w240) -> ()
                        n217 = local write "MFLI-1-Settings"(w240) -> ()
                      }
                      frame "2" {
                        n218 = local read "MFLI-1-Settings"() -> (w245:T1)
                        n219 = Bundle By Name(cluster=w245, "Demod 2 Osc"=w244) -> (w243:T1)
                        n220 = global write "Instrument_Setup.vi" "MFLI-1-Settings"(w243) -> ()
                        n221 = local write "MFLI-1-Settings"(w243) -> ()
                      }
                      frame "3" {
                        n222 = local read "MFLI-1-Settings"() -> (w248:T1)
                        n223 = Bundle By Name(cluster=w248, "Demod 3 Osc"=w247) -> (w246:T1)
                        n224 = global write "Instrument_Setup.vi" "MFLI-1-Settings"(w246) -> ()
                        n225 = local write "MFLI-1-Settings"(w246) -> ()
                      }
                    }
                  }
                  frame "HARMONIC" {
                    n226 = call-poly "ziGetEvent.vi"("Handle In"=w254) -> ("Sample Out"=w253:T6, "Handle Out"=w249:T4)  [unwired: 8 in, 1 out]
                    n227 = Unbundle(w253) -> ("Value"=w252:i64[])  [unwired: 1 out]
                    n228 = Index Array(array=w252) -> (element=w251:i64)  [unwired: 1 in]
                    n229 = case shown="\"3\"" w250 {
                      tunnel: w251 -> [_ w256 w259 w262 w265]
                      frame Default {
                      }
                      frame "0" {
                        n230 = local read "MFLI-1-Settings"() -> (w257:T1)
                        n231 = Bundle By Name(cluster=w257, "Demod 0 Harm"=w256) -> (w255:T1)
                        n232 = global write "Instrument_Setup.vi" "MFLI-1-Settings"(w255) -> ()
                        n233 = local write "MFLI-1-Settings"(w255) -> ()
                      }
                      frame "1" {
                        n234 = local read "MFLI-1-Settings"() -> (w260:T1)
                        n235 = Bundle By Name(cluster=w260, "Demod 1 Harm"=w259) -> (w258:T1)
                        n236 = local write "MFLI-1-Settings"(w258) -> ()
                        n237 = global write "Instrument_Setup.vi" "MFLI-1-Settings"(w258) -> ()
                      }
                      frame "2" {
                        n238 = local read "MFLI-1-Settings"() -> (w263:T1)
                        n239 = Bundle By Name(cluster=w263, "Demod 2 Harm"=w262) -> (w261:T1)
                        n240 = global write "Instrument_Setup.vi" "MFLI-1-Settings"(w261) -> ()
                        n241 = local write "MFLI-1-Settings"(w261) -> ()
                      }
                      frame "3" {
                        n242 = local read "MFLI-1-Settings"() -> (w266:T1)
                        n243 = Bundle By Name(cluster=w266, "Demod 3 Harm"=w265) -> (w264:T1)
                        n244 = global write "Instrument_Setup.vi" "MFLI-1-Settings"(w264) -> ()
                        n245 = local write "MFLI-1-Settings"(w264) -> ()
                      }
                    }
                  }
                  frame "PHASESHIFT" {
                    n246 = call-poly "ziGetEvent.vi"("Handle In"=w272) -> ("Sample Out"=w270:T5, "Handle Out"=w267:T4)  [unwired: 8 in, 1 out]
                    n247 = Unbundle(w270) -> ("Value"=w269:dbl[])  [unwired: 1 out]
                    n248 = Index Array(array=w269) -> (element=w268:dbl)  [unwired: 1 in]
                    n249 = case shown="\"0\"" w271 {
                      tunnel: w268 -> [_ w274 w277 w280 w283]
                      frame Default {
                      }
                      frame "0" {
                        n250 = local read "MFLI-1-Settings"() -> (w275:T1)
                        n251 = Bundle By Name(cluster=w275, "Demod 0 Phase"=w274) -> (w273:T1)
                        n252 = local write "MFLI-1-Settings"(w273) -> ()
                        n253 = global write "Instrument_Setup.vi" "MFLI-1-Settings"(w273) -> ()
                      }
                      frame "1" {
                        n254 = local read "MFLI-1-Settings"() -> (w278:T1)
                        n255 = Bundle By Name(cluster=w278, "Demod 1 Phase"=w277) -> (w276:T1)
                        n256 = global write "Instrument_Setup.vi" "MFLI-1-Settings"(w276) -> ()
                        n257 = local write "MFLI-1-Settings"(w276) -> ()
                      }
                      frame "2" {
                        n258 = local read "MFLI-1-Settings"() -> (w281:T1)
                        n259 = Bundle By Name(cluster=w281, "Demod 2 Phase"=w280) -> (w279:T1)
                        n260 = global write "Instrument_Setup.vi" "MFLI-1-Settings"(w279) -> ()
                        n261 = local write "MFLI-1-Settings"(w279) -> ()
                      }
                      frame "3" {
                        n262 = local read "MFLI-1-Settings"() -> (w284:T1)
                        n263 = Bundle By Name(cluster=w284, "Demod 3 Phase"=w283) -> (w282:T1)
                        n264 = global write "Instrument_Setup.vi" "MFLI-1-Settings"(w282) -> ()
                        n265 = local write "MFLI-1-Settings"(w282) -> ()
                      }
                    }
                  }
                  frame "ADCSELECT" {
                    n266 = call-poly "ziGetEvent.vi"("Handle In"=w290) -> ("Sample Out"=w289:T6, "Handle Out"=w285:T4)  [unwired: 8 in, 1 out]
                    n267 = Unbundle(w289) -> ("Value"=w288:i64[])  [unwired: 1 out]
                    n268 = Index Array(array=w288) -> (element=w286:i64)  [unwired: 1 in]
                    n269 = case shown="\"2\"" w287 {
                      tunnel: w286 -> [_ w294 w298 w302 w306]
                      frame Default {
                      }
                      frame "0" {
                        n270 = Number To Decimal String(number=w294) -> (decimal integer string=w292:string)  [unwired: 1 in]
                        n271 = local read "MFLI-1-Settings"() -> (w293:T1)
                        n272 = Bundle By Name(cluster=w293, "Input Demod 0"=w292) -> (w291:T1)
                        n273 = local write "MFLI-1-Settings"(w291) -> ()
                        n274 = global write "Instrument_Setup.vi" "MFLI-1-Settings"(w291) -> ()
                      }
                      frame "1" {
                        n275 = Number To Decimal String(number=w298) -> (decimal integer string=w296:string)  [unwired: 1 in]
                        n276 = local read "MFLI-1-Settings"() -> (w297:T1)
                        n277 = Bundle By Name(cluster=w297, "Input Demod 1"=w296) -> (w295:T1)
                        n278 = global write "Instrument_Setup.vi" "MFLI-1-Settings"(w295) -> ()
                        n279 = local write "MFLI-1-Settings"(w295) -> ()
                      }
                      frame "2" {
                        n280 = Number To Decimal String(number=w302) -> (decimal integer string=w300:string)  [unwired: 1 in]
                        n281 = local read "MFLI-1-Settings"() -> (w301:T1)
                        n282 = Bundle By Name(cluster=w301, "Input Demod 2"=w300) -> (w299:T1)
                        n283 = local write "MFLI-1-Settings"(w299) -> ()
                        n284 = global write "Instrument_Setup.vi" "MFLI-1-Settings"(w299) -> ()
                      }
                      frame "3" {
                        n285 = Number To Decimal String(number=w306) -> (decimal integer string=w304:string)  [unwired: 1 in]
                        n286 = local read "MFLI-1-Settings"() -> (w305:T1)
                        n287 = Bundle By Name(cluster=w305, "Input Demod 3"=w304) -> (w303:T1)
                        n288 = global write "Instrument_Setup.vi" "MFLI-1-Settings"(w303) -> ()
                        n289 = local write "MFLI-1-Settings"(w303) -> ()
                      }
                    }
                  }
                  frame "ORDER" {
                    n290 = call-poly "ziGetEvent.vi"("Handle In"=w312) -> ("Sample Out"=w310:T6, "Handle Out"=w307:T4)  [unwired: 8 in, 1 out]
                    n291 = Unbundle(w310) -> ("Value"=w309:i64[])  [unwired: 1 out]
                    n292 = Index Array(array=w309) -> (element=w308:i64)  [unwired: 1 in]
                    n293 = case shown="\"0\"" w311 {
                      tunnel: w308 -> [_ w314 w317 w320 w323]
                      frame Default {
                      }
                      frame "0" {
                        n294 = local read "MFLI-1-Settings"() -> (w315:T1)
                        n295 = Bundle By Name(cluster=w315, "Demod 0 Order"=w314) -> (w313:T1)
                        n296 = local write "MFLI-1-Settings"(w313) -> ()
                        n297 = global write "Instrument_Setup.vi" "MFLI-1-Settings"(w313) -> ()
                      }
                      frame "1" {
                        n298 = local read "MFLI-1-Settings"() -> (w318:T1)
                        n299 = Bundle By Name(cluster=w318, "Demod 1 Order"=w317) -> (w316:T1)
                        n300 = global write "Instrument_Setup.vi" "MFLI-1-Settings"(w316) -> ()
                        n301 = local write "MFLI-1-Settings"(w316) -> ()
                      }
                      frame "2" {
                        n302 = local read "MFLI-1-Settings"() -> (w321:T1)
                        n303 = Bundle By Name(cluster=w321, "Demod 2 Order"=w320) -> (w319:T1)
                        n304 = local write "MFLI-1-Settings"(w319) -> ()
                        n305 = global write "Instrument_Setup.vi" "MFLI-1-Settings"(w319) -> ()
                      }
                      frame "3" {
                        n306 = local read "MFLI-1-Settings"() -> (w324:T1)
                        n307 = Bundle By Name(cluster=w324, "Demod 3 Order"=w323) -> (w322:T1)
                        n308 = local write "MFLI-1-Settings"(w322) -> ()
                        n309 = global write "Instrument_Setup.vi" "MFLI-1-Settings"(w322) -> ()
                      }
                    }
                  }
                  frame "TIMECONSTANT" {
                    n310 = call-poly "ziGetEvent.vi"("Handle In"=w330) -> ("Sample Out"=w329:T5, "Handle Out"=w325:T4)  [unwired: 8 in, 1 out]
                    n311 = Unbundle(w329) -> ("Value"=w328:dbl[])  [unwired: 1 out]
                    n312 = Index Array(array=w328) -> (element=w326:dbl)  [unwired: 1 in]
                    n313 = case shown="\"2\"" w327 {
                      tunnel: w326 -> [_ w332 w335 w338 w341]
                      frame Default {
                      }
                      frame "0" {
                        n314 = local read "MFLI-1-Settings"() -> (w333:T1)
                        n315 = Bundle By Name(cluster=w333, "Demod 0 TC"=w332) -> (w331:T1)
                        n316 = global write "Instrument_Setup.vi" "MFLI-1-Settings"(w331) -> ()
                        n317 = local write "MFLI-1-Settings"(w331) -> ()
                      }
                      frame "1" {
                        n318 = local read "MFLI-1-Settings"() -> (w336:T1)
                        n319 = Bundle By Name(cluster=w336, "Demod 1 TC"=w335) -> (w334:T1)
                        n320 = global write "Instrument_Setup.vi" "MFLI-1-Settings"(w334) -> ()
                        n321 = local write "MFLI-1-Settings"(w334) -> ()
                      }
                      frame "2" {
                        n322 = local read "MFLI-1-Settings"() -> (w339:T1)
                        n323 = Bundle By Name(cluster=w339, "Demod 2 TC"=w338) -> (w337:T1)
                        n324 = global write "Instrument_Setup.vi" "MFLI-1-Settings"(w337) -> ()
                        n325 = local write "MFLI-1-Settings"(w337) -> ()
                      }
                      frame "3" {
                        n326 = local read "MFLI-1-Settings"() -> (w342:T1)
                        n327 = Bundle By Name(cluster=w342, "Demod 3 TC"=w341) -> (w340:T1)
                        n328 = global write "Instrument_Setup.vi" "MFLI-1-Settings"(w340) -> ()
                        n329 = local write "MFLI-1-Settings"(w340) -> ()
                      }
                    }
                  }
                  frame "SINC" {
                    n330 = call-poly "ziGetEvent.vi"("Handle In"=w344) -> ("Sample Out"=w349:T6, "Handle Out"=w343:T4)  [unwired: 8 in, 1 out]
                    n331 = Unbundle(w349) -> ("Value"=w348:i64[])  [unwired: 1 out]
                    n332 = Index Array(array=w348) -> (element=w346:i64)  [unwired: 1 in]
                    n333 = Not Equal To 0?(x=w346) -> (x != 0?=w345:bool)
                    n334 = case shown="\"0\"" w347 {
                      tunnel: w345 -> [_ w351 w354 w357 w360]
                      frame Default {
                      }
                      frame "0" {
                        n335 = local read "MFLI-1-Settings"() -> (w352:T1)
                        n336 = Bundle By Name(cluster=w352, "Demod 0 Sinc"=w351) -> (w350:T1)
                        n337 = local write "MFLI-1-Settings"(w350) -> ()
                        n338 = global write "Instrument_Setup.vi" "MFLI-1-Settings"(w350) -> ()
                      }
                      frame "1" {
                        n339 = local read "MFLI-1-Settings"() -> (w355:T1)
                        n340 = Bundle By Name(cluster=w355, "Demod 1 Sinc"=w354) -> (w353:T1)
                        n341 = local write "MFLI-1-Settings"(w353) -> ()
                        n342 = global write "Instrument_Setup.vi" "MFLI-1-Settings"(w353) -> ()
                      }
                      frame "2" {
                        n343 = local read "MFLI-1-Settings"() -> (w358:T1)
                        n344 = Bundle By Name(cluster=w358, "Demod 2 Sinc"=w357) -> (w356:T1)
                        n345 = global write "Instrument_Setup.vi" "MFLI-1-Settings"(w356) -> ()
                        n346 = local write "MFLI-1-Settings"(w356) -> ()
                      }
                      frame "3" {
                        n347 = local read "MFLI-1-Settings"() -> (w361:T1)
                        n348 = Bundle By Name(cluster=w361, "Demod 3 Sinc"=w360) -> (w359:T1)
                        n349 = local write "MFLI-1-Settings"(w359) -> ()
                        n350 = global write "Instrument_Setup.vi" "MFLI-1-Settings"(w359) -> ()
                      }
                    }
                  }
                  frame "ENABLE" {
                    n351 = call-poly "ziGetEvent.vi"("Handle In"=w369) -> ("Sample Out"=w368:T6, "Handle Out"=w363:T4)  [unwired: 8 in, 1 out]
                    n352 = Unbundle(w368) -> ("Value"=w367:i64[])  [unwired: 1 out]
                    n353 = Index Array(array=w367) -> (element=w366:i64)  [unwired: 1 in]
                    n354 = Not Equal To 0?(x=w366) -> (x != 0?=w365:bool)
                    n355 = case shown="\"0\"" w364 {
                      tunnel: w365 -> [_ w372 w384 w396 w408]
                      tunnel: w363 -> [w370 w376 w387 w398 w411]
                      tunnel: [w370 w375 w386 w399 w410] -> w362
                      frame Default {
                      }
                      frame "0" {
                        n356 = local read "MFLI-1-Settings"() -> (w373:T1)
                        n357 = Bundle By Name(cluster=w373, "Demod 0 Enable"=w372) -> (w371:T1)
                        n358 = global write "Instrument_Setup.vi" "MFLI-1-Settings"(w371) -> ()
                        n359 = local write "MFLI-1-Settings"(w371) -> ()
                        n360 = case shown="False" w372 {
                          tunnel: w376 -> [w379 w382]
                          tunnel: [w378 w381] -> w375
                          tunnel: "demods/0/sample" ("Path ()") -> [w377 w380]
                          frame False {
                            n361 = call "ziUnSubscribe.vi"("Path (\"/\")"=w377, "Handle in"=w379) -> ("Handle out"=w378:T4)  [unwired: 2 in, 1 out]
                          }
                          frame True {
                            n362 = call "ziSubscribe.vi"("Path ()"=w380, "Handle In"=w382) -> ("Handle Out"=w381:T4)  [unwired: 2 in, 1 out]
                          }
                        }
                      }
                      frame "1" {
                        n363 = local read "MFLI-1-Settings"() -> (w385:T1)
                        n364 = Bundle By Name(cluster=w385, "Demod 1 Enable"=w384) -> (w383:T1)
                        n365 = global write "Instrument_Setup.vi" "MFLI-1-Settings"(w383) -> ()
                        n366 = local write "MFLI-1-Settings"(w383) -> ()
                        n367 = case shown="True" w384 {
                          tunnel: w387 -> [w391 w394]
                          tunnel: [w390 w393] -> w386
                          tunnel: "demods/1/sample" ("Path ()") -> [w389 w392]
                          frame False {
                            n368 = call "ziUnSubscribe.vi"("Path (\"/\")"=w389, "Handle in"=w391) -> ("Handle out"=w390:T4)  [unwired: 2 in, 1 out]
                          }
                          frame True {
                            n369 = call "ziSubscribe.vi"("Path ()"=w392, "Handle In"=w394) -> ("Handle Out"=w393:T4)  [unwired: 2 in, 1 out]
                          }
                        }
                      }
                      frame "2" {
                        n370 = local read "MFLI-1-Settings"() -> (w397:T1)
                        n371 = Bundle By Name(cluster=w397, "Demod 2 Enable"=w396) -> (w395:T1)
                        n372 = global write "Instrument_Setup.vi" "MFLI-1-Settings"(w395) -> ()
                        n373 = local write "MFLI-1-Settings"(w395) -> ()
                        n374 = case shown="False" w396 {
                          tunnel: w398 -> [w403 w406]
                          tunnel: [w402 w405] -> w399
                          tunnel: "demods/2/sample" ("Path ()") -> [w401 w404]
                          frame False {
                            n375 = call "ziUnSubscribe.vi"("Path (\"/\")"=w401, "Handle in"=w403) -> ("Handle out"=w402:T4)  [unwired: 2 in, 1 out]
                          }
                          frame True {
                            n376 = call "ziSubscribe.vi"("Path ()"=w404, "Handle In"=w406) -> ("Handle Out"=w405:T4)  [unwired: 2 in, 1 out]
                          }
                        }
                      }
                      frame "3" {
                        n377 = local read "MFLI-1-Settings"() -> (w409:T1)
                        n378 = Bundle By Name(cluster=w409, "Demod 3 Enable"=w408) -> (w407:T1)
                        n379 = local write "MFLI-1-Settings"(w407) -> ()
                        n380 = global write "Instrument_Setup.vi" "MFLI-1-Settings"(w407) -> ()
                        n381 = case shown="True" w408 {
                          tunnel: w411 -> [w415 w418]
                          tunnel: [w414 w417] -> w410
                          tunnel: "demods/3/sample" ("Path ()") -> [w413 w416]
                          frame False {
                            n382 = call "ziUnSubscribe.vi"("Path (\"/\")"=w413, "Handle in"=w415) -> ("Handle out"=w414:T4)  [unwired: 2 in, 1 out]
                          }
                          frame True {
                            n383 = call "ziSubscribe.vi"("Path ()"=w416, "Handle In"=w418) -> ("Handle Out"=w417:T4)  [unwired: 2 in, 1 out]
                          }
                        }
                      }
                    }
                  }
                  frame "RATE" {
                    n384 = call-poly "ziGetEvent.vi"("Handle In"=w424) -> ("Sample Out"=w423:T5, "Handle Out"=w419:T4)  [unwired: 8 in, 1 out]
                    n385 = Unbundle(w423) -> ("Value"=w422:dbl[])  [unwired: 1 out]
                    n386 = Index Array(array=w422) -> (element=w420:dbl)  [unwired: 1 in]
                    n387 = case shown="\"0\"" w421 {
                      tunnel: w420 -> [_ w426 w429 w432 w435]
                      frame Default {
                      }
                      frame "0" {
                        n388 = local read "MFLI-1-Settings"() -> (w427:T1)
                        n389 = Bundle By Name(cluster=w427, "Demod 0 Data Rate"=w426) -> (w425:T1)
                        n390 = local write "MFLI-1-Settings"(w425) -> ()
                        n391 = global write "Instrument_Setup.vi" "MFLI-1-Settings"(w425) -> ()
                      }
                      frame "1" {
                        n392 = local read "MFLI-1-Settings"() -> (w430:T1)
                        n393 = Bundle By Name(cluster=w430, "Demod 1 Data Rate"=w429) -> (w428:T1)
                        n394 = global write "Instrument_Setup.vi" "MFLI-1-Settings"(w428) -> ()
                        n395 = local write "MFLI-1-Settings"(w428) -> ()
                      }
                      frame "2" {
                        n396 = local read "MFLI-1-Settings"() -> (w433:T1)
                        n397 = Bundle By Name(cluster=w433, "Demod 2 Data Rate"=w432) -> (w431:T1)
                        n398 = local write "MFLI-1-Settings"(w431) -> ()
                        n399 = global write "Instrument_Setup.vi" "MFLI-1-Settings"(w431) -> ()
                      }
                      frame "3" {
                        n400 = local read "MFLI-1-Settings"() -> (w436:T1)
                        n401 = Bundle By Name(cluster=w436, "Demod 3 Data Rate"=w435) -> (w434:T1)
                        n402 = local write "MFLI-1-Settings"(w434) -> ()
                        n403 = global write "Instrument_Setup.vi" "MFLI-1-Settings"(w434) -> ()
                      }
                    }
                  }
                  frame "SAMPLE" {
                    n404 = call-poly "ziGetEvent.vi"("Handle In"=w445) -> ("Demod Sample Out"=w441:T3, "Handle Out"=w440:T4)  [unwired: 8 in, 1 out]
                    n405 = Unbundle(w441) -> ("X (Vrms)"=w437:dbl[], "Y (Vrms)"=w438:dbl[])  [unwired: 7 out]
                    n406 = Build Array(w437, w438) -> (w443:dbl[][])
                    n407 = Transpose 2D Array(2D array=w443) -> (transposed array=w442:dbl[][])
                    n408 = case shown="\"1\"" w444 {
                      tunnel: w442 -> [_ w448 w459 w469 w479]
                      tunnel: w441 -> [_ w449 w458 w468 w478]
                      tunnel: w439 -> [_ _ _ _ _]
                      tunnel: w438 -> [_ w447 w457 w467 w477]
                      tunnel: w437 -> [_ w446 w456 w466 w476]
                      frame Default {
                      }
                      frame "0" {
                        n409 = for {
                          tunnel: w447 -> [w454] mode=indexing
                          tunnel: w446 -> [w453] mode=indexing
                          n410 = local read "MFL_Monitor"() -> (w455:T2)
                          n411 = Bundle By Name(cluster=w455, "Demod 0 :X"=w453, "Demod 0 :Y"=w454) -> (w452:T2)
                          n412 = local write "MFL_Monitor"(w452) -> ()
                        }
                        n413 = local read "MFL_Monitor"() -> (w451:T2)
                        n414 = Bundle By Name(cluster=w451, "Demod 0"=w448, "Demod Sample out 0"=w449) -> (w450:T2)
                        n415 = local write "MFL_Monitor"(w450) -> ()
                      }
                      frame "1" {
                        n416 = for {
                          tunnel: w457 -> [w464] mode=indexing
                          tunnel: w456 -> [w463] mode=indexing
                          n417 = local read "MFL_Monitor"() -> (w465:T2)
                          n418 = Bundle By Name(cluster=w465, "Demod 1 :X"=w463, "Demod 1 :Y"=w464) -> (w462:T2)
                          n419 = local write "MFL_Monitor"(w462) -> ()
                        }
                        n420 = local read "MFL_Monitor"() -> (w461:T2)
                        n421 = Bundle By Name(cluster=w461, "Demod 1"=w459, "Demod Sample out 1"=w458) -> (w460:T2)
                        n422 = local write "MFL_Monitor"(w460) -> ()
                      }
                      frame "2" {
                        n423 = for {
                          tunnel: w467 -> [w473] mode=indexing
                          tunnel: w466 -> [w472] mode=indexing
                          n424 = local read "MFL_Monitor"() -> (w475:T2)
                          n425 = Bundle By Name(cluster=w475, "Demod 2 :X"=w472, "Demod 2 :Y"=w473) -> (w474:T2)
                          n426 = local write "MFL_Monitor"(w474) -> ()
                        }
                        n427 = local read "MFL_Monitor"() -> (w471:T2)
                        n428 = Bundle By Name(cluster=w471, "Demod 2"=w469, "Demod Sample out 2"=w468) -> (w470:T2)
                        n429 = local write "MFL_Monitor"(w470) -> ()
                      }
                      frame "3" {
                        n430 = for {
                          tunnel: w477 -> [w483] mode=indexing
                          tunnel: w476 -> [w482] mode=indexing
                          n431 = local read "MFL_Monitor"() -> (w485:T2)
                          n432 = Bundle By Name(cluster=w485, "Demod 3 :X"=w482, "Demod 3 :Y"=w483) -> (w484:T2)
                          n433 = local write "MFL_Monitor"(w484) -> ()
                        }
                        n434 = local read "MFL_Monitor"() -> (w481:T2)
                        n435 = Bundle By Name(cluster=w481, "Demod 3"=w479, "Demod Sample out 3"=w478) -> (w480:T2)
                        n436 = local write "MFL_Monitor"(w480) -> ()
                      }
                    }
                  }
                }
              }
              frame "AUXOUTS" {
                n437 = case shown="\"PREOFFSET\"" w489 {
                  tunnel: w488 -> [_ w492 w511 w529 w547 w565]
                  tunnel: w487 -> [w490 w497 w515 w533 w551 w569]
                  tunnel: [w490 w496 w514 w532 w550 w568] -> w486
                  frame Default {
                  }
                  frame "OUTPUTSELECT" {
                    n438 = call-poly "ziGetEvent.vi"("Handle In"=w497) -> ("Sample Out"=w495:T6, "Handle Out"=w496:T4)  [unwired: 8 in, 1 out]
                    n439 = Unbundle(w495) -> ("Value"=w494:i64[])  [unwired: 1 out]
                    n440 = Index Array(array=w494) -> (element=w493:i64)  [unwired: 1 in]
                    n441 = Number To Decimal String(number=w493) -> (decimal integer string=w491:string)  [unwired: 1 in]
                    n442 = case shown="Default" w492 {
                      tunnel: w491 -> [_ w499 w502 w505 w508]
                      frame Default {
                      }
                      frame "0" {
                        n443 = local read "MFLI-1-Settings"() -> (w500:T1)
                        n444 = Bundle By Name(cluster=w500, "Aux Out 0 Select"=w499) -> (w498:T1)
                        n445 = local write "MFLI-1-Settings"(w498) -> ()
                        n446 = global write "Instrument_Setup.vi" "MFLI-1-Settings"(w498) -> ()
                      }
                      frame "1" {
                        n447 = local read "MFLI-1-Settings"() -> (w503:T1)
                        n448 = Bundle By Name(cluster=w503, "Aux Out 1 Select"=w502) -> (w501:T1)
                        n449 = global write "Instrument_Setup.vi" "MFLI-1-Settings"(w501) -> ()
                        n450 = local write "MFLI-1-Settings"(w501) -> ()
                      }
                      frame "2" {
                        n451 = local read "MFLI-1-Settings"() -> (w506:T1)
                        n452 = Bundle By Name(cluster=w506, "Aux Out 2 Select"=w505) -> (w504:T1)
                        n453 = global write "Instrument_Setup.vi" "MFLI-1-Settings"(w504) -> ()
                        n454 = local write "MFLI-1-Settings"(w504) -> ()
                      }
                      frame "3" {
                        n455 = local read "MFLI-1-Settings"() -> (w509:T1)
                        n456 = Bundle By Name(cluster=w509, "Aux Out 3 Select"=w508) -> (w507:T1)
                        n457 = local write "MFLI-1-Settings"(w507) -> ()
                        n458 = global write "Instrument_Setup.vi" "MFLI-1-Settings"(w507) -> ()
                      }
                    }
                  }
                  frame "DEMODSELECT" {
                    n459 = call-poly "ziGetEvent.vi"("Handle In"=w515) -> ("Sample Out"=w513:T6, "Handle Out"=w514:T4)  [unwired: 8 in, 1 out]
                    n460 = Unbundle(w513) -> ("Value"=w512:i64[])  [unwired: 1 out]
                    n461 = Index Array(array=w512) -> (element=w510:i64)  [unwired: 1 in]
                    n462 = case shown="\"3\"" w511 {
                      tunnel: w510 -> [_ w517 w520 w523 w526]
                      frame Default {
                      }
                      frame "0" {
                        n463 = local read "MFLI-1-Settings"() -> (w518:T1)
                        n464 = Bundle By Name(cluster=w518, "Aux Out 0 Demod Num"=w517) -> (w516:T1)
                        n465 = local write "MFLI-1-Settings"(w516) -> ()
                        n466 = global write "Instrument_Setup.vi" "MFLI-1-Settings"(w516) -> ()
                      }
                      frame "1" {
                        n467 = local read "MFLI-1-Settings"() -> (w521:T1)
                        n468 = Bundle By Name(cluster=w521, "Aux Out 1 Demod Num"=w520) -> (w519:T1)
                        n469 = local write "MFLI-1-Settings"(w519) -> ()
                        n470 = global write "Instrument_Setup.vi" "MFLI-1-Settings"(w519) -> ()
                      }
                      frame "2" {
                        n471 = local read "MFLI-1-Settings"() -> (w524:T1)
                        n472 = Bundle By Name(cluster=w524, "Aux Out 2 Demod Num"=w523) -> (w522:T1)
                        n473 = local write "MFLI-1-Settings"(w522) -> ()
                        n474 = global write "Instrument_Setup.vi" "MFLI-1-Settings"(w522) -> ()
                      }
                      frame "3" {
                        n475 = local read "MFLI-1-Settings"() -> (w527:T1)
                        n476 = Bundle By Name(cluster=w527, "Aux Out 3 Demod Num"=w526) -> (w525:T1)
                        n477 = local write "MFLI-1-Settings"(w525) -> ()
                        n478 = global write "Instrument_Setup.vi" "MFLI-1-Settings"(w525) -> ()
                      }
                    }
                  }
                  frame "PREOFFSET" {
                    n479 = call-poly "ziGetEvent.vi"("Handle In"=w533) -> ("Sample Out"=w531:T5, "Handle Out"=w532:T4)  [unwired: 8 in, 1 out]
                    n480 = Unbundle(w531) -> ("Value"=w530:dbl[])  [unwired: 1 out]
                    n481 = Index Array(array=w530) -> (element=w528:dbl)  [unwired: 1 in]
                    n482 = case shown="\"0\"" w529 {
                      tunnel: w528 -> [_ w535 w538 w541 w544]
                      frame Default {
                      }
                      frame "0" {
                        n483 = local read "MFLI-1-Settings"() -> (w536:T1)
                        n484 = Bundle By Name(cluster=w536, "Aux Out 0 Pre Offset"=w535) -> (w534:T1)
                        n485 = local write "MFLI-1-Settings"(w534) -> ()
                        n486 = global write "Instrument_Setup.vi" "MFLI-1-Settings"(w534) -> ()
                      }
                      frame "1" {
                        n487 = local read "MFLI-1-Settings"() -> (w539:T1)
                        n488 = Bundle By Name(cluster=w539, "Aux Out 1 Pre Offset"=w538) -> (w537:T1)
                        n489 = local write "MFLI-1-Settings"(w537) -> ()
                        n490 = global write "Instrument_Setup.vi" "MFLI-1-Settings"(w537) -> ()
                      }
                      frame "2" {
                        n491 = local read "MFLI-1-Settings"() -> (w542:T1)
                        n492 = Bundle By Name(cluster=w542, "Aux Out 2 Pre Offset"=w541) -> (w540:T1)
                        n493 = local write "MFLI-1-Settings"(w540) -> ()
                        n494 = global write "Instrument_Setup.vi" "MFLI-1-Settings"(w540) -> ()
                      }
                      frame "3" {
                        n495 = local read "MFLI-1-Settings"() -> (w545:T1)
                        n496 = Bundle By Name(cluster=w545, "Aux Out 3 Pre Offset"=w544) -> (w543:T1)
                        n497 = local write "MFLI-1-Settings"(w543) -> ()
                        n498 = global write "Instrument_Setup.vi" "MFLI-1-Settings"(w543) -> ()
                      }
                    }
                  }
                  frame "SCALE" {
                    n499 = call-poly "ziGetEvent.vi"("Handle In"=w551) -> ("Sample Out"=w549:T5, "Handle Out"=w550:T4)  [unwired: 8 in, 1 out]
                    n500 = Unbundle(w549) -> ("Value"=w548:dbl[])  [unwired: 1 out]
                    n501 = Index Array(array=w548) -> (element=w546:dbl)  [unwired: 1 in]
                    n502 = case shown="\"1\"" w547 {
                      tunnel: w546 -> [_ w553 w556 w559 w562]
                      frame Default {
                      }
                      frame "0" {
                        n503 = local read "MFLI-1-Settings"() -> (w554:T1)
                        n504 = Bundle By Name(cluster=w554, "Aux Out 0 Scale"=w553) -> (w552:T1)
                        n505 = global write "Instrument_Setup.vi" "MFLI-1-Settings"(w552) -> ()
                        n506 = local write "MFLI-1-Settings"(w552) -> ()
                      }
                      frame "1" {
                        n507 = local read "MFLI-1-Settings"() -> (w557:T1)
                        n508 = Bundle By Name(cluster=w557, "Aux Out 1 Scale"=w556) -> (w555:T1)
                        n509 = local write "MFLI-1-Settings"(w555) -> ()
                        n510 = global write "Instrument_Setup.vi" "MFLI-1-Settings"(w555) -> ()
                      }
                      frame "2" {
                        n511 = local read "MFLI-1-Settings"() -> (w560:T1)
                        n512 = Bundle By Name(cluster=w560, "Aux Out 2 Scale"=w559) -> (w558:T1)
                        n513 = local write "MFLI-1-Settings"(w558) -> ()
                        n514 = global write "Instrument_Setup.vi" "MFLI-1-Settings"(w558) -> ()
                      }
                      frame "3" {
                        n515 = local read "MFLI-1-Settings"() -> (w563:T1)
                        n516 = Bundle By Name(cluster=w563, "Aux Out 3 Scale"=w562) -> (w561:T1)
                        n517 = local write "MFLI-1-Settings"(w561) -> ()
                        n518 = global write "Instrument_Setup.vi" "MFLI-1-Settings"(w561) -> ()
                      }
                    }
                  }
                  frame "OFFSET" {
                    n519 = call-poly "ziGetEvent.vi"("Handle In"=w569) -> ("Sample Out"=w567:T5, "Handle Out"=w568:T4)  [unwired: 8 in, 1 out]
                    n520 = Unbundle(w567) -> ("Value"=w566:dbl[])  [unwired: 1 out]
                    n521 = Index Array(array=w566) -> (element=w564:dbl)  [unwired: 1 in]
                    n522 = case shown="Default" w565 {
                      tunnel: w564 -> [_ w571 w574 w577 w580]
                      frame Default {
                      }
                      frame "0" {
                        n523 = local read "MFLI-1-Settings"() -> (w572:T1)
                        n524 = Bundle By Name(cluster=w572, "Aux Out 0 Offset"=w571) -> (w570:T1)
                        n525 = local write "MFLI-1-Settings"(w570) -> ()
                        n526 = global write "Instrument_Setup.vi" "MFLI-1-Settings"(w570) -> ()
                      }
                      frame "1" {
                        n527 = local read "MFLI-1-Settings"() -> (w575:T1)
                        n528 = Bundle By Name(cluster=w575, "Aux Out 1 Offset"=w574) -> (w573:T1)
                        n529 = local write "MFLI-1-Settings"(w573) -> ()
                        n530 = global write "Instrument_Setup.vi" "MFLI-1-Settings"(w573) -> ()
                      }
                      frame "2" {
                        n531 = local read "MFLI-1-Settings"() -> (w578:T1)
                        n532 = Bundle By Name(cluster=w578, "Aux Out 2 Offset"=w577) -> (w576:T1)
                        n533 = local write "MFLI-1-Settings"(w576) -> ()
                        n534 = global write "Instrument_Setup.vi" "MFLI-1-Settings"(w576) -> ()
                      }
                      frame "3" {
                        n535 = local read "MFLI-1-Settings"() -> (w581:T1)
                        n536 = Bundle By Name(cluster=w581, "Aux Out 3 Offset"=w580) -> (w579:T1)
                        n537 = local write "MFLI-1-Settings"(w579) -> ()
                        n538 = global write "Instrument_Setup.vi" "MFLI-1-Settings"(w579) -> ()
                      }
                    }
                  }
                }
              }
            }
          }
          frame #1 {
            n539 = global read "Instrument_Setup.vi" "MFLI-1-Settings"() -> (w585:T1)
            n540 = local read "MFLI-1-Settings"() -> (w586:T1)
            n541 = global read "Instrument_Setup.vi" "Update Lockins"() -> (w583:bool)
            n542 = Equal?(x=w586, y=w585) -> (x = y?=w588:T7)
            n543 = Cluster To Array(cluster=w588) -> (array=w587:bool[])
            n544 = And Array Elements(Boolean array=w587) -> (logical AND=w584:bool)
            n545 = And(x=w584, y=w583) -> (x .and. y?=w582:bool)
          }
          frame #2 {
            n546 = call "MFL_Open_Queue.vi"() -> ("queue out"=w593:refnum<queue>)  [unwired: 10 in, 1 out]
            n547 = call "MFL_Check_Queue.vi"("queue"=w593) -> ("MFL_Monitor"=w592:T2, "New Entries?"=w591:bool)  [unwired: 3 in, 1 out]
            "Value in Queue" <- w591
          }
          frame #3 {
            n548 = Or(x=w597, y=w595) -> (x .or. y?=w596:bool)
            n549 = case shown="True" w596 {
              tunnel: w600 -> [w601 w605]
              tunnel: [w601 w604] -> w599
              tunnel: w598 -> [_ w603]
              tunnel: w595 -> [_ w602]
              frame False {
              }
              frame True {
                n550 = stacked-sequence {
                  seq-local: [w610 _ _ _ _ _] -> [_ _ w1041 _ _ _]
                  seq-local: [_ _ w1037 _ _ _] -> [_ _ _ w1065 _ _]
                  seq-local: [_ _ _ w1064 _ _] -> [_ _ _ _ w1091 _]
                  seq-local: [_ _ _ _ w1090 _] -> [_ _ _ _ _ w1146]
                  tunnel: w605 -> [w611 _ _ _ _ _]
                  tunnel: [_ _ _ _ _ w1132] -> w604
                  tunnel: w603 -> [w609 _ w1036 w1063 w1089 w1150]
                  tunnel: w602 -> [w606 _ _ _ _ _]
                  frame #0 {
                    n551 = Unbundle By Name(w609) -> ("Update Lock-In"=w608:bool)
                    n552 = Or(x=w608, y=w606) -> (x .or. y?=w607:bool)
                    n553 = case shown="True" w607 {
                      tunnel: w611 -> [w612 w616]
                      tunnel: [w612 w615] -> w610
                      frame False {
                      }
                      frame True {
                        n554 = flat-sequence {
                          tunnel: w616 -> [w618]
                          tunnel: [w618] -> w614
                          tunnel: w614 -> [w620]
                          tunnel: [w619] -> w613
                          tunnel: [w1022] -> w615
                          tunnel: w613 -> [w1022]
                          frame #0 {
                            n555 = global read "Instrument_Setup.vi" "MFLI-1-Settings"() -> (w617:T1)
                            n556 = local write "MFLI-1-Settings"(w617) -> ()
                          }
                          frame #1 {
                            n557 = event shown="[52] \"MFLI-1-Settings.Add\": Value Change" {
                              selector: _ -> [_ _ _ _ _ _ _ _ _ _ _ _ _ _ _ _ _ _ _ _ _ _ _ _ _ _ _ _ _ _ _ _ _ _ _ _ _ _ _ _ _ _ _ _ _ _ _ _ _ _ _ _ _ _ _ _ _ _ _ _ _ _ _ _ _ _ _ _ _ _ _ _ _ _ _]
                              dyn-events: _ -> [_ _ _ _ _ _ _ _ _ _ _ _ _ _ _ _ _ _ _ _ _ _ _ _ _ _ _ _ _ _ _ _ _ _ _ _ _ _ _ _ _ _ _ _ _ _ _ _ _ _ _ _ _ _ _ _ _ _ _ _ _ _ _ _ _ _ _ _ _ _ _ _ _ _ _]
                              timeout: _ -> [_ _ _ _ _ _ _ _ _ _ _ _ _ _ _ _ _ _ _ _ _ _ _ _ _ _ _ _ _ _ _ _ _ _ _ _ _ _ _ _ _ _ _ _ _ _ _ _ _ _ _ _ _ _ _ _ _ _ _ _ _ _ _ _ _ _ _ _ _ _ _ _ _ _ _]
                              tunnel: w620 -> [w625 w629 w635 w640 w645 w650 w655 w660 w665 w670 w675 w680 w685 w690 w695 w700 w706 w711 w716 w722 w728 w733 w738 w744 w749 w753 w759 w764 w770 w776 w781 w788 w794 w799 w804 w812 w816 w822 w827 w831 w837 w841 w846 w852 w858 w864 w869 w876 w882 w888 w893 w899 w905 w911 w915 w920 w926 w932 w938 w944 w949 w954 w959 w964 w969 w974 w979 w984 w989 w994 w999 w1004 w1009 w1014 w1019]
                              tunnel: [w624 w628 w634 w639 w644 w649 w654 w659 w664 w669 w674 w679 w684 w689 w694 w699 w705 w710 w715 w721 w727 w732 w737 w743 w748 w752 w758 w763 w769 w775 w780 w787 w793 w798 w803 w811 w815 w821 w826 w830 w836 w840 w845 w851 w857 w863 w868 w875 w881 w887 w892 w898 w904 w910 w914 w919 w925 w931 w937 w943 w948 w953 w958 w963 w968 w973 w978 w983 w988 w993 w998 w1003 w1008 w1013 w1018] -> w619
                              event Value Change {
                                n558 = event-data() -> ()  [unwired: 1 in, 5 out]
                                n559 = local read "MFLI-1-Settings"() -> (w622:T1)
                                n560 = Unbundle By Name(w622) -> ("Osc 0 Freq"=w621:dbl)
                                n561 = call-poly "ziSetValue.vi"("Value"=w621, "Path"="oscs/0/freq", "Handle In"=w625) -> ("Handle Out"=w624:T4)  [unwired: 2 in, 1 out]
                              }
                              event Value Change {
                                n562 = event-data() -> ()  [unwired: 1 in, 6 out]
                                n563 = local read "MFLI-1-Settings"() -> (w627:T1)
                                n564 = Unbundle By Name(w627) -> ("Osc 1 Freq"=w626:dbl)
                                n565 = call-poly "ziSetValue.vi"("Value"=w626, "Path"="oscs/1/freq", "Handle In"=w629) -> ("Handle Out"=w628:T4)  [unwired: 2 in, 1 out]
                              }
                              event Value Change {
                                n566 = event-data() -> ()  [unwired: 1 in, 6 out]
                                n567 = local read "MFLI-1-Settings"() -> (w632:T1)
                                n568 = Unbundle By Name(w632) -> ("Osc 2 Freq"=w631:dbl)
                                n569 = call-poly "ziSetValue.vi"("Value"=w631, "Path"="oscs/2/freq", "Handle In"=w635) -> ("Handle Out"=w634:T4)  [unwired: 2 in, 1 out]
                              }
                              event Value Change {
                                n570 = event-data() -> ()  [unwired: 1 in, 6 out]
                                n571 = local read "MFLI-1-Settings"() -> (w637:T1)
                                n572 = Unbundle By Name(w637) -> ("Osc 3 Freq"=w636:dbl)
                                n573 = call-poly "ziSetValue.vi"("Value"=w636, "Path"="oscs/3/freq", "Handle In"=w640) -> ("Handle Out"=w639:T4)  [unwired: 2 in, 1 out]
                              }
                              event Value Change {
                                n574 = event-data() -> ()  [unwired: 1 in, 6 out]
                                n575 = local read "MFLI-1-Settings"() -> (w642:T1)
                                n576 = Unbundle By Name(w642) -> ("Demod 0 Osc"=w641:i8)
                                n577 = call-poly "ziSetValue.vi"("Value"=w641, "Path"="demods/0/oscselect", "Handle In"=w645) -> ("Handle Out"=w644:T4)  [unwired: 2 in, 1 out]
                              }
                              event Value Change {
                                n578 = event-data() -> ()  [unwired: 1 in, 6 out]
                                n579 = local read "MFLI-1-Settings"() -> (w647:T1)
                                n580 = Unbundle By Name(w647) -> ("Demod 1 Osc"=w646:i8)
                                n581 = call-poly "ziSetValue.vi"("Value"=w646, "Path"="demods/1/oscselect", "Handle In"=w650) -> ("Handle Out"=w649:T4)  [unwired: 2 in, 1 out]
                              }
                              event Value Change {
                                n582 = event-data() -> ()  [unwired: 1 in, 6 out]
                                n583 = local read "MFLI-1-Settings"() -> (w652:T1)
                                n584 = Unbundle By Name(w652) -> ("Demod 2 Osc"=w651:i8)
                                n585 = call-poly "ziSetValue.vi"("Value"=w651, "Path"="demods/2/oscselect", "Handle In"=w655) -> ("Handle Out"=w654:T4)  [unwired: 2 in, 1 out]
                              }
                              event Value Change {
                                n586 = event-data() -> ()  [unwired: 1 in, 6 out]
                                n587 = local read "MFLI-1-Settings"() -> (w657:T1)
                                n588 = Unbundle By Name(w657) -> ("Demod 3 Osc"=w656:i8)
                                n589 = call-poly "ziSetValue.vi"("Value"=w656, "Path"="demods/3/oscselect", "Handle In"=w660) -> ("Handle Out"=w659:T4)  [unwired: 2 in, 1 out]
                              }
                              event Value Change {
                                n590 = event-data() -> ()  [unwired: 1 in, 6 out]
                                n591 = local read "MFLI-1-Settings"() -> (w662:T1)
                                n592 = Unbundle By Name(w662) -> ("Demod 0 Harm"=w661:i16)
                                n593 = call-poly "ziSetValue.vi"("Value"=w661, "Path"="demods/0/harmonic", "Handle In"=w665) -> ("Handle Out"=w664:T4)  [unwired: 2 in, 1 out]
                              }
                              event Value Change {
                                n594 = event-data() -> ()  [unwired: 1 in, 6 out]
                                n595 = local read "MFLI-1-Settings"() -> (w667:T1)
                                n596 = Unbundle By Name(w667) -> ("Demod 0 Phase"=w666:dbl)
                                n597 = call-poly "ziSetValue.vi"("Value"=w666, "Path"="demods/0/phaseshift", "Handle In"=w670) -> ("Handle Out"=w669:T4)  [unwired: 2 in, 1 out]
                              }
                              event Value Change {
                                n598 = event-data() -> ()  [unwired: 1 in, 6 out]
                                n599 = local read "MFLI-1-Settings"() -> (w672:T1)
                                n600 = Unbundle By Name(w672) -> ("Demod 1 Phase"=w671:dbl)
                                n601 = call-poly "ziSetValue.vi"("Value"=w671, "Path"="demods/1/phaseshift", "Handle In"=w675) -> ("Handle Out"=w674:T4)  [unwired: 2 in, 1 out]
                              }
                              event Value Change {
                                n602 = event-data() -> ()  [unwired: 1 in, 6 out]
                                n603 = local read "MFLI-1-Settings"() -> (w677:T1)
                                n604 = Unbundle By Name(w677) -> ("Demod 2 Phase"=w676:dbl)
                                n605 = call-poly "ziSetValue.vi"("Value"=w676, "Path"="demods/2/phaseshift", "Handle In"=w680) -> ("Handle Out"=w679:T4)  [unwired: 2 in, 1 out]
                              }
                              event Value Change {
                                n606 = event-data() -> ()  [unwired: 1 in, 6 out]
                                n607 = local read "MFLI-1-Settings"() -> (w682:T1)
                                n608 = Unbundle By Name(w682) -> ("Demod 3 Phase"=w681:dbl)
                                n609 = call-poly "ziSetValue.vi"("Value"=w681, "Path"="demods/3/phaseshift", "Handle In"=w685) -> ("Handle Out"=w684:T4)  [unwired: 2 in, 1 out]
                              }
                              event Value Change {
                                n610 = event-data() -> ()  [unwired: 1 in, 6 out]
                                n611 = local read "MFLI-1-Settings"() -> (w687:T1)
                                n612 = Unbundle By Name(w687) -> ("Demod 1 Harm"=w686:i16)
                                n613 = call-poly "ziSetValue.vi"("Value"=w686, "Path"="demods/1/harmonic", "Handle In"=w690) -> ("Handle Out"=w689:T4)  [unwired: 2 in, 1 out]
                              }
                              event Value Change {
                                n614 = event-data() -> ()  [unwired: 1 in, 6 out]
                                n615 = local read "MFLI-1-Settings"() -> (w692:T1)
                                n616 = Unbundle By Name(w692) -> ("Demod 2 Harm"=w691:i16)
                                n617 = call-poly "ziSetValue.vi"("Value"=w691, "Path"="demods/2/harmonic", "Handle In"=w695) -> ("Handle Out"=w694:T4)  [unwired: 2 in, 1 out]
                              }
                              event Value Change {
                                n618 = event-data() -> ()  [unwired: 1 in, 6 out]
                                n619 = local read "MFLI-1-Settings"() -> (w697:T1)
                                n620 = Unbundle By Name(w697) -> ("Demod 3 Harm"=w696:i16)
                                n621 = call-poly "ziSetValue.vi"("Value"=w696, "Path"="demods/3/harmonic", "Handle In"=w700) -> ("Handle Out"=w699:T4)  [unwired: 2 in, 1 out]
                              }
                              event Value Change {
                                n622 = event-data() -> ()  [unwired: 1 in, 6 out]
                                n623 = local read "MFLI-1-Settings"() -> (w702:T1)
                                n624 = Unbundle By Name(w702) -> ("Input Demod 0"=w701:string)
                                n625 = Decimal String To Number(string=w701) -> (number=w703:i32)  [unwired: 2 in, 1 out]
                                n626 = call-poly "ziSetValue.vi"("Value"=w703, "Path"="demods/0/adcselect", "Handle In"=w706) -> ("Handle Out"=w705:T4)  [unwired: 2 in, 1 out]
                              }
                              event Value Change {
                                n627 = event-data() -> ()  [unwired: 1 in, 6 out]
                                n628 = local read "MFLI-1-Settings"() -> (w708:T1)
                                n629 = Unbundle By Name(w708) -> ("Input Demod 1"=w707:string)
                                n630 = Decimal String To Number(string=w707) -> (number=w712:i32)  [unwired: 2 in, 1 out]
                                n631 = call-poly "ziSetValue.vi"("Value"=w712, "Path"="demods/1/adcselect", "Handle In"=w711) -> ("Handle Out"=w710:T4)  [unwired: 2 in, 1 out]
                              }
                              event Value Change {
                                n632 = event-data() -> ()  [unwired: 1 in, 6 out]
                                n633 = local read "MFLI-1-Settings"() -> (w714:T1)
                                n634 = Unbundle By Name(w714) -> ("Input Demod 2"=w713:string)
                                n635 = Decimal String To Number(string=w713) -> (number=w718:i32)  [unwired: 2 in, 1 out]
                                n636 = call-poly "ziSetValue.vi"("Value"=w718, "Path"="demods/2/adcselect", "Handle In"=w716) -> ("Handle Out"=w715:T4)  [unwired: 2 in, 1 out]
                              }
                              event Value Change {
                                n637 = event-data() -> ()  [unwired: 1 in, 6 out]
                                n638 = local read "MFLI-1-Settings"() -> (w720:T1)
                                n639 = Unbundle By Name(w720) -> ("Input Demod 3"=w719:string)
                                n640 = Decimal String To Number(string=w719) -> (number=w724:i32)  [unwired: 2 in, 1 out]
                                n641 = call-poly "ziSetValue.vi"("Value"=w724, "Path"="demods/3/adcselect", "Handle In"=w722) -> ("Handle Out"=w721:T4)  [unwired: 2 in, 1 out]
                              }
                              event Value Change {
                                n642 = event-data() -> ()  [unwired: 1 in, 6 out]
                                n643 = local read "MFLI-1-Settings"() -> (w726:T1)
                                n644 = Unbundle By Name(w726) -> ("Demod 0 Order"=w725:i8)
                                n645 = call-poly "ziSetValue.vi"("Value"=w725, "Path"="demods/0/order", "Handle In"=w728) -> ("Handle Out"=w727:T4)  [unwired: 2 in, 1 out]
                              }
                              event Value Change {
                                n646 = event-data() -> ()  [unwired: 1 in, 6 out]
                                n647 = local read "MFLI-1-Settings"() -> (w731:T1)
                                n648 = Unbundle By Name(w731) -> ("Demod 1 Order"=w730:i8)
                                n649 = call-poly "ziSetValue.vi"("Value"=w730, "Path"="demods/1/order", "Handle In"=w733) -> ("Handle Out"=w732:T4)  [unwired: 2 in, 1 out]
                              }
                              event Value Change {
                                n650 = event-data() -> ()  [unwired: 1 in, 6 out]
                                n651 = local read "MFLI-1-Settings"() -> (w736:T1)
                                n652 = Unbundle By Name(w736) -> ("Demod 2 Order"=w735:i8)
                                n653 = call-poly "ziSetValue.vi"("Value"=w735, "Path"="demods/2/order", "Handle In"=w738) -> ("Handle Out"=w737:T4)  [unwired: 2 in, 1 out]
                              }
                              event Value Change {
                                n654 = event-data() -> ()  [unwired: 1 in, 6 out]
                                n655 = local read "MFLI-1-Settings"() -> (w741:T1)
                                n656 = Unbundle By Name(w741) -> ("Demod 3 Order"=w740:i8)
                                n657 = call-poly "ziSetValue.vi"("Value"=w740, "Path"="demods/3/order", "Handle In"=w744) -> ("Handle Out"=w743:T4)  [unwired: 2 in, 1 out]
                              }
                              event Value Change {
                                n658 = event-data() -> ()  [unwired: 1 in, 6 out]
                                n659 = local read "MFLI-1-Settings"() -> (w746:T1)
                                n660 = Unbundle By Name(w746) -> ("Demod 0 TC"=w745:dbl)
                                n661 = call-poly "ziSetValue.vi"("Value"=w745, "Path"="demods/0/timeconstant", "Handle In"=w749) -> ("Handle Out"=w748:T4)  [unwired: 2 in, 1 out]
                              }
                              event Value Change {
                                n662 = event-data() -> ()  [unwired: 1 in, 6 out]
                                n663 = local read "MFLI-1-Settings"() -> (w751:T1)
                                n664 = Unbundle By Name(w751) -> ("Demod 1 TC"=w750:dbl)
                                n665 = call-poly "ziSetValue.vi"("Value"=w750, "Path"="demods/1/timeconstant", "Handle In"=w753) -> ("Handle Out"=w752:T4)  [unwired: 2 in, 1 out]
                              }
                              event Value Change {
                                n666 = event-data() -> ()  [unwired: 1 in, 6 out]
                                n667 = local read "MFLI-1-Settings"() -> (w756:T1)
                                n668 = Unbundle By Name(w756) -> ("Demod 2 TC"=w755:dbl)
                                n669 = call-poly "ziSetValue.vi"("Value"=w755, "Path"="demods/2/timeconstant", "Handle In"=w759) -> ("Handle Out"=w758:T4)  [unwired: 2 in, 1 out]
                              }
                              event Value Change {
                                n670 = event-data() -> ()  [unwired: 1 in, 6 out]
                                n671 = local read "MFLI-1-Settings"() -> (w761:T1)
                                n672 = Unbundle By Name(w761) -> ("Demod 3 TC"=w760:dbl)
                                n673 = call-poly "ziSetValue.vi"("Value"=w760, "Path"="demods/3/timeconstant", "Handle In"=w764) -> ("Handle Out"=w763:T4)  [unwired: 2 in, 1 out]
                              }
                              event Value Change {
                                n674 = event-data() -> ()  [unwired: 1 in, 6 out]
                                n675 = local read "MFLI-1-Settings"() -> (w766:T1)
                                n676 = Unbundle By Name(w766) -> ("Demod 0 Sinc"=w765:bool)
                                n677 = Boolean To (0,1)(Boolean=w765) -> (0, 1=w767:i16)
                                n678 = call-poly "ziSetValue.vi"("Value"=w767, "Path"="demods/0/sinc", "Handle In"=w770) -> ("Handle Out"=w769:T4)  [unwired: 2 in, 1 out]
                              }
                              event Value Change {
                                n679 = event-data() -> ()  [unwired: 1 in, 6 out]
                                n680 = local read "MFLI-1-Settings"() -> (w772:T1)
                                n681 = Unbundle By Name(w772) -> ("Demod 1 Sinc"=w771:bool)
                                n682 = Boolean To (0,1)(Boolean=w771) -> (0, 1=w773:i16)
                                n683 = call-poly "ziSetValue.vi"("Value"=w773, "Path"="demods/1/sinc", "Handle In"=w776) -> ("Handle Out"=w775:T4)  [unwired: 2 in, 1 out]
                              }
                              event Value Change {
                                n684 = event-data() -> ()  [unwired: 1 in, 6 out]
                                n685 = local read "MFLI-1-Settings"() -> (w778:T1)
                                n686 = Unbundle By Name(w778) -> ("Demod 2 Sinc"=w777:bool)
                                n687 = Boolean To (0,1)(Boolean=w777) -> (0, 1=w782:i16)
                                n688 = call-poly "ziSetValue.vi"("Value"=w782, "Path"="demods/2/sinc", "Handle In"=w781) -> ("Handle Out"=w780:T4)  [unwired: 2 in, 1 out]
                              }
                              event Value Change {
                                n689 = event-data() -> ()  [unwired: 1 in, 6 out]
                                n690 = local read "MFLI-1-Settings"() -> (w784:T1)
                                n691 = Unbundle By Name(w784) -> ("Demod 3 Sinc"=w783:bool)
                                n692 = Boolean To (0,1)(Boolean=w783) -> (0, 1=w785:i16)
                                n693 = call-poly "ziSetValue.vi"("Value"=w785, "Path"="demods/3/sinc", "Handle In"=w788) -> ("Handle Out"=w787:T4)  [unwired: 2 in, 1 out]
                              }
                              event Value Change {
                                n694 = event-data() -> ()  [unwired: 1 in, 6 out]
                                n695 = local read "MFLI-1-Settings"() -> (w790:T1)
                                n696 = Unbundle By Name(w790) -> ("Demod 0 Enable"=w789:bool)
                                n697 = Boolean To (0,1)(Boolean=w789) -> (0, 1=w791:i16)
                                n698 = call-poly "ziSetValue.vi"("Value"=w791, "Path"="demods/0/enable", "Handle In"=w794) -> ("Handle Out"=w793:T4)  [unwired: 2 in, 1 out]
                              }
                              event Value Change {
                                n699 = event-data() -> ()  [unwired: 1 in, 6 out]
                                n700 = local read "MFLI-1-Settings"() -> (w796:T1)
                                n701 = Unbundle By Name(w796) -> ("Demod 1 Enable"=w795:bool)
                                n702 = Boolean To (0,1)(Boolean=w795) -> (0, 1=w797:i16)
                                n703 = call-poly "ziSetValue.vi"("Value"=w797, "Path"="demods/1/enable", "Handle In"=w799) -> ("Handle Out"=w798:T4)  [unwired: 2 in, 1 out]
                              }
                              event Value Change {
                                n704 = event-data() -> ()  [unwired: 1 in, 6 out]
                                n705 = local read "MFLI-1-Settings"() -> (w802:T1)
                                n706 = Unbundle By Name(w802) -> ("Demod 2 Enable"=w801:bool)
                                n707 = Boolean To (0,1)(Boolean=w801) -> (0, 1=w806:i16)
                                n708 = call-poly "ziSetValue.vi"("Value"=w806, "Path"="demods/2/enable", "Handle In"=w804) -> ("Handle Out"=w803:T4)  [unwired: 2 in, 1 out]
                              }
                              event Value Change {
                                n709 = event-data() -> ()  [unwired: 1 in, 6 out]
                                n710 = local read "MFLI-1-Settings"() -> (w808:T1)
                                n711 = Unbundle By Name(w808) -> ("Demod 3 Enable"=w807:bool)
                                n712 = Boolean To (0,1)(Boolean=w807) -> (0, 1=w809:i16)
                                n713 = call-poly "ziSetValue.vi"("Value"=w809, "Path"="demods/3/enable", "Handle In"=w812) -> ("Handle Out"=w811:T4)  [unwired: 2 in, 1 out]
                              }
                              event Value Change {
                                n714 = event-data() -> ()  [unwired: 1 in, 6 out]
                                n715 = local read "MFLI-1-Settings"() -> (w814:T1)
                                n716 = Unbundle By Name(w814) -> ("Demod 0 Data Rate"=w813:dbl)
                                n717 = call-poly "ziSetValue.vi"("Value"=w813, "Path"="demods/0/rate", "Handle In"=w816) -> ("Handle Out"=w815:T4)  [unwired: 2 in, 1 out]
                              }
                              event Value Change {
                                n718 = event-data() -> ()  [unwired: 1 in, 6 out]
                                n719 = local read "MFLI-1-Settings"() -> (w819:T1)
                                n720 = Unbundle By Name(w819) -> ("Demod 1 Data Rate"=w818:dbl)
                                n721 = call-poly "ziSetValue.vi"("Value"=w818, "Path"="demods/1/rate", "Handle In"=w822) -> ("Handle Out"=w821:T4)  [unwired: 2 in, 1 out]
                              }
                              event Value Change {
                                n722 = event-data() -> ()  [unwired: 1 in, 6 out]
                                n723 = local read "MFLI-1-Settings"() -> (w824:T1)
                                n724 = Unbundle By Name(w824) -> ("Demod 2 Data Rate"=w823:dbl)
                                n725 = call-poly "ziSetValue.vi"("Value"=w823, "Path"="demods/2/rate", "Handle In"=w827) -> ("Handle Out"=w826:T4)  [unwired: 2 in, 1 out]
                              }
                              event Value Change {
                                n726 = event-data() -> ()  [unwired: 1 in, 6 out]
                                n727 = local read "MFLI-1-Settings"() -> (w829:T1)
                                n728 = Unbundle By Name(w829) -> ("Demod 3 Data Rate"=w828:dbl)
                                n729 = call-poly "ziSetValue.vi"("Value"=w828, "Path"="demods/3/rate", "Handle In"=w831) -> ("Handle Out"=w830:T4)  [unwired: 2 in, 1 out]
                              }
                              event Value Change {
                                n730 = event-data() -> ()  [unwired: 1 in, 6 out]
                                n731 = local read "MFLI-1-Settings"() -> (w834:T1)
                                n732 = Unbundle By Name(w834) -> ("Ampl 0"=w833:dbl)
                                n733 = call-poly "ziSetValue.vi"("Value"=w833, "Path"="sigouts/0/amplitudes/0", "Handle In"=w837) -> ("Handle Out"=w836:T4)  [unwired: 2 in, 1 out]
                              }
                              event Value Change {
                                n734 = event-data() -> ()  [unwired: 1 in, 6 out]
                                n735 = local read "MFLI-1-Settings"() -> (w839:T1)
                                n736 = Unbundle By Name(w839) -> ("Ampl 1"=w838:dbl)
                                n737 = call-poly "ziSetValue.vi"("Value"=w838, "Path"="sigouts/0/amplitudes/1", "Handle In"=w841) -> ("Handle Out"=w840:T4)  [unwired: 2 in, 1 out]
                              }
                              event Value Change {
                                n738 = event-data() -> ()  [unwired: 1 in, 6 out]
                                n739 = local read "MFLI-1-Settings"() -> (w844:T1)
                                n740 = Unbundle By Name(w844) -> ("Ampl 2"=w843:dbl)
                                n741 = call-poly "ziSetValue.vi"("Value"=w843, "Path"="sigouts/0/amplitudes/2", "Handle In"=w846) -> ("Handle Out"=w845:T4)  [unwired: 2 in, 1 out]
                              }
                              event Value Change {
                                n742 = event-data() -> ()  [unwired: 1 in, 6 out]
                                n743 = local read "MFLI-1-Settings"() -> (w849:T1)
                                n744 = Unbundle By Name(w849) -> ("Ampl 3"=w848:dbl)
                                n745 = call-poly "ziSetValue.vi"("Value"=w848, "Path"="sigouts/0/amplitudes/3", "Handle In"=w852) -> ("Handle Out"=w851:T4)  [unwired: 2 in, 1 out]
                              }
                              event Value Change {
                                n746 = event-data() -> ()  [unwired: 1 in, 6 out]
                                n747 = local read "MFLI-1-Settings"() -> (w854:T1)
                                n748 = Unbundle By Name(w854) -> ("Ampl 0 Enable"=w853:bool)
                                n749 = Boolean To (0,1)(Boolean=w853) -> (0, 1=w855:i16)
                                n750 = call-poly "ziSetValue.vi"("Value"=w855, "Path"="sigouts/0/enables/0", "Handle In"=w858) -> ("Handle Out"=w857:T4)  [unwired: 2 in, 1 out]
                              }
                              event Value Change {
                                n751 = event-data() -> ()  [unwired: 1 in, 6 out]
                                n752 = local read "MFLI-1-Settings"() -> (w860:T1)
                                n753 = Unbundle By Name(w860) -> ("Ampl 1 Enable"=w859:bool)
                                n754 = Boolean To (0,1)(Boolean=w859) -> (0, 1=w861:i16)
                                n755 = call-poly "ziSetValue.vi"("Value"=w861, "Path"="sigouts/0/enables/1", "Handle In"=w864) -> ("Handle Out"=w863:T4)  [unwired: 2 in, 1 out]
                              }
                              event Value Change {
                                n756 = event-data() -> ()  [unwired: 1 in, 6 out]
                                n757 = local read "MFLI-1-Settings"() -> (w866:T1)
                                n758 = Unbundle By Name(w866) -> ("Ampl 3 Enable"=w865:bool)
                                n759 = Boolean To (0,1)(Boolean=w865) -> (0, 1=w867:i16)
                                n760 = call-poly "ziSetValue.vi"("Value"=w867, "Path"="sigouts/0/enables/3", "Handle In"=w869) -> ("Handle Out"=w868:T4)  [unwired: 2 in, 1 out]
                              }
                              event Value Change {
                                n761 = event-data() -> ()  [unwired: 1 in, 6 out]
                                n762 = local read "MFLI-1-Settings"() -> (w872:T1)
                                n763 = Unbundle By Name(w872) -> ("Ampl 2 Enable"=w871:bool)
                                n764 = Boolean To (0,1)(Boolean=w871) -> (0, 1=w874:i16)
                                n765 = call-poly "ziSetValue.vi"("Value"=w874, "Path"="sigouts/0/enables/2", "Handle In"=w876) -> ("Handle Out"=w875:T4)  [unwired: 2 in, 1 out]
                              }
                              event Value Change {
                                n766 = event-data() -> ()  [unwired: 1 in, 6 out]
                                n767 = local read "MFLI-1-Settings"() -> (w878:T1)
                                n768 = Unbundle By Name(w878) -> ("On"=w877:bool)
                                n769 = Boolean To (0,1)(Boolean=w877) -> (0, 1=w879:i16)
                                n770 = call-poly "ziSetValue.vi"("Value"=w879, "Path"="sigouts/0/on", "Handle In"=w882) -> ("Handle Out"=w881:T4)  [unwired: 2 in, 1 out]
                              }
                              event Value Change {
                                n771 = event-data() -> ()  [unwired: 1 in, 6 out]
                                n772 = local read "MFLI-1-Settings"() -> (w884:T1)
                                n773 = Unbundle By Name(w884) -> ("50 Ohm"=w883:bool)
                                n774 = Boolean To (0,1)(Boolean=w883) -> (0, 1=w885:i16)
                                n775 = call-poly "ziSetValue.vi"("Value"=w885, "Path"="sigouts/0/imp50", "Handle In"=w888) -> ("Handle Out"=w887:T4)  [unwired: 2 in, 1 out]
                              }
                              event Value Change {
                                n776 = event-data() -> ()  [unwired: 1 in, 6 out]
                                n777 = local read "MFLI-1-Settings"() -> (w890:T1)
                                n778 = Unbundle By Name(w890) -> ("Range (V)"=w889:dbl)
                                n779 = call-poly "ziSetValue.vi"("Value"=w889, "Path"="sigouts/0/range", "Handle In"=w893) -> ("Handle Out"=w892:T4)  [unwired: 2 in, 1 out]
                              }
                              event Value Change {
                                n780 = event-data() -> ()  [unwired: 1 in, 6 out]
                                n781 = local read "MFLI-1-Settings"() -> (w895:T1)
                                n782 = Unbundle By Name(w895) -> ("Auto-Range"=w894:bool)
                                n783 = Boolean To (0,1)(Boolean=w894) -> (0, 1=w897:i16)
                                n784 = call-poly "ziSetValue.vi"("Value"=w897, "Path"="sigouts/0/autorange", "Handle In"=w899) -> ("Handle Out"=w898:T4)  [unwired: 2 in, 1 out]
                              }
                              event Value Change {
                                n785 = event-data() -> ()  [unwired: 1 in, 6 out]
                                n786 = local read "MFLI-1-Settings"() -> (w901:T1)
                                n787 = Unbundle By Name(w901) -> ("Add"=w900:bool)
                                n788 = Boolean To (0,1)(Boolean=w900) -> (0, 1=w903:i16)
                                n789 = call-poly "ziSetValue.vi"("Value"=w903, "Path"="sigouts/0/add", "Handle In"=w905) -> ("Handle Out"=w904:T4)  [unwired: 2 in, 1 out]
                              }
                              event Value Change {
                                n790 = event-data() -> ()  [unwired: 1 in, 6 out]
                                n791 = local read "MFLI-1-Settings"() -> (w907:T1)
                                n792 = Unbundle By Name(w907) -> ("Diff"=w906:bool)
                                n793 = Boolean To (0,1)(Boolean=w906) -> (0, 1=w908:i16)
                                n794 = call-poly "ziSetValue.vi"("Value"=w908, "Path"="sigouts/0/diff", "Handle In"=w911) -> ("Handle Out"=w910:T4)  [unwired: 2 in, 1 out]
                              }
                              event Value Change {
                                n795 = event-data() -> ()  [unwired: 1 in, 6 out]
                                n796 = local read "MFLI-1-Settings"() -> (w913:T1)
                                n797 = Unbundle By Name(w913) -> ("Offset (V)"=w912:dbl)
                                n798 = call-poly "ziSetValue.vi"("Value"=w912, "Path"="sigouts/0/offset", "Handle In"=w915) -> ("Handle Out"=w914:T4)  [unwired: 2 in, 1 out]
                              }
                              event Value Change {
                                n799 = event-data() -> ()  [unwired: 1 in, 6 out]
                                n800 = local read "MFLI-1-Settings"() -> (w918:T1)
                                n801 = Unbundle By Name(w918) -> ("Aux Out 0 Select"=w917:string)
                                n802 = Decimal String To Number(string=w917) -> (number=w921:i32)  [unwired: 2 in, 1 out]
                                n803 = call-poly "ziSetValue.vi"("Value"=w921, "Path"="auxouts/0/outputselect", "Handle In"=w920) -> ("Handle Out"=w919:T4)  [unwired: 2 in, 1 out]
                              }
                              event Value Change {
                                n804 = event-data() -> ()  [unwired: 1 in, 6 out]
                                n805 = local read "MFLI-1-Settings"() -> (w924:T1)
                                n806 = Unbundle By Name(w924) -> ("Aux Out 1 Select"=w923:string)
                                n807 = Decimal String To Number(string=w923) -> (number=w928:i32)  [unwired: 2 in, 1 out]
                                n808 = call-poly "ziSetValue.vi"("Value"=w928, "Path"="auxouts/1/outputselect", "Handle In"=w926) -> ("Handle Out"=w925:T4)  [unwired: 2 in, 1 out]
                              }
                              event Value Change {
                                n809 = event-data() -> ()  [unwired: 1 in, 6 out]
                                n810 = local read "MFLI-1-Settings"() -> (w930:T1)
                                n811 = Unbundle By Name(w930) -> ("Aux Out 2 Select"=w929:string)
                                n812 = Decimal String To Number(string=w929) -> (number=w934:i32)  [unwired: 2 in, 1 out]
                                n813 = call-poly "ziSetValue.vi"("Value"=w934, "Path"="auxouts/2/outputselect", "Handle In"=w932) -> ("Handle Out"=w931:T4)  [unwired: 2 in, 1 out]
                              }
                              event Value Change {
                                n814 = event-data() -> ()  [unwired: 1 in, 6 out]
                                n815 = local read "MFLI-1-Settings"() -> (w936:T1)
                                n816 = Unbundle By Name(w936) -> ("Aux Out 3 Select"=w935:string)
                                n817 = Decimal String To Number(string=w935) -> (number=w940:i32)  [unwired: 2 in, 1 out]
                                n818 = call-poly "ziSetValue.vi"("Value"=w940, "Path"="auxouts/3/outputselect", "Handle In"=w938) -> ("Handle Out"=w937:T4)  [unwired: 2 in, 1 out]
                              }
                              event Value Change {
                                n819 = event-data() -> ()  [unwired: 1 in, 6 out]
                                n820 = local read "MFLI-1-Settings"() -> (w942:T1)
                                n821 = Unbundle By Name(w942) -> ("Aux Out 0 Demod Num"=w941:dbl)
                                n822 = call-poly "ziSetValue.vi"("Value"=w941, "Path"="auxouts/0/demodselect", "Handle In"=w944) -> ("Handle Out"=w943:T4)  [unwired: 2 in, 1 out]
                              }
                              event Value Change {
                                n823 = event-data() -> ()  [unwired: 1 in, 6 out]
                                n824 = local read "MFLI-1-Settings"() -> (w947:T1)
                                n825 = Unbundle By Name(w947) -> ("Aux Out 1 Demod Num"=w946:dbl)
                                n826 = call-poly "ziSetValue.vi"("Value"=w946, "Path"="auxouts/1/demodselect", "Handle In"=w949) -> ("Handle Out"=w948:T4)  [unwired: 2 in, 1 out]
                              }
                              event Value Change {
                                n827 = event-data() -> ()  [unwired: 1 in, 6 out]
                                n828 = local read "MFLI-1-Settings"() -> (w952:T1)
                                n829 = Unbundle By Name(w952) -> ("Aux Out 2 Demod Num"=w951:dbl)
                                n830 = call-poly "ziSetValue.vi"("Value"=w951, "Path"="auxouts/2/demodselect", "Handle In"=w954) -> ("Handle Out"=w953:T4)  [unwired: 2 in, 1 out]
                              }
                              event Value Change {
                                n831 = event-data() -> ()  [unwired: 1 in, 6 out]
                                n832 = local read "MFLI-1-Settings"() -> (w957:T1)
                                n833 = Unbundle By Name(w957) -> ("Aux Out 3 Demod Num"=w956:dbl)
                                n834 = call-poly "ziSetValue.vi"("Value"=w956, "Path"="auxouts/3/demodselect", "Handle In"=w959) -> ("Handle Out"=w958:T4)  [unwired: 2 in, 1 out]
                              }
                              event Value Change {
                                n835 = event-data() -> ()  [unwired: 1 in, 6 out]
                                n836 = local read "MFLI-1-Settings"() -> (w962:T1)
                                n837 = Unbundle By Name(w962) -> ("Aux Out 0 Pre Offset"=w961:dbl)
                                n838 = call-poly "ziSetValue.vi"("Value"=w961, "Path"="auxouts/0/preoffset", "Handle In"=w964) -> ("Handle Out"=w963:T4)  [unwired: 2 in, 1 out]
                              }
                              event Value Change {
                                n839 = event-data() -> ()  [unwired: 1 in, 6 out]
                                n840 = local read "MFLI-1-Settings"() -> (w967:T1)
                                n841 = Unbundle By Name(w967) -> ("Aux Out 1 Pre Offset"=w966:dbl)
                                n842 = call-poly "ziSetValue.vi"("Value"=w966, "Path"="auxouts/1/preoffset", "Handle In"=w969) -> ("Handle Out"=w968:T4)  [unwired: 2 in, 1 out]
                              }
                              event Value Change {
                                n843 = event-data() -> ()  [unwired: 1 in, 6 out]
                                n844 = local read "MFLI-1-Settings"() -> (w972:T1)
                                n845 = Unbundle By Name(w972) -> ("Aux Out 2 Pre Offset"=w971:dbl)
                                n846 = call-poly "ziSetValue.vi"("Value"=w971, "Path"="auxouts/2/preoffset", "Handle In"=w974) -> ("Handle Out"=w973:T4)  [unwired: 2 in, 1 out]
                              }
                              event Value Change {
                                n847 = event-data() -> ()  [unwired: 1 in, 6 out]
                                n848 = local read "MFLI-1-Settings"() -> (w977:T1)
                                n849 = Unbundle By Name(w977) -> ("Aux Out 3 Pre Offset"=w976:dbl)
                                n850 = call-poly "ziSetValue.vi"("Value"=w976, "Path"="auxouts/3/preoffset", "Handle In"=w979) -> ("Handle Out"=w978:T4)  [unwired: 2 in, 1 out]
                              }
                              event Value Change {
                                n851 = event-data() -> ()  [unwired: 1 in, 6 out]
                                n852 = local read "MFLI-1-Settings"() -> (w982:T1)
                                n853 = Unbundle By Name(w982) -> ("Aux Out 0 Scale"=w981:dbl)
                                n854 = call-poly "ziSetValue.vi"("Value"=w981, "Path"="auxouts/0/scale", "Handle In"=w984) -> ("Handle Out"=w983:T4)  [unwired: 2 in, 1 out]
                              }
                              event Value Change {
                                n855 = event-data() -> ()  [unwired: 1 in, 6 out]
                                n856 = local read "MFLI-1-Settings"() -> (w987:T1)
                                n857 = Unbundle By Name(w987) -> ("Aux Out 1 Scale"=w986:dbl)
                                n858 = call-poly "ziSetValue.vi"("Value"=w986, "Path"="auxouts/1/scale", "Handle In"=w989) -> ("Handle Out"=w988:T4)  [unwired: 2 in, 1 out]
                              }
                              event Value Change {
                                n859 = event-data() -> ()  [unwired: 1 in, 6 out]
                                n860 = local read "MFLI-1-Settings"() -> (w992:T1)
                                n861 = Unbundle By Name(w992) -> ("Aux Out 2 Scale"=w991:dbl)
                                n862 = call-poly "ziSetValue.vi"("Value"=w991, "Path"="auxouts/2/scale", "Handle In"=w994) -> ("Handle Out"=w993:T4)  [unwired: 2 in, 1 out]
                              }
                              event Value Change {
                                n863 = event-data() -> ()  [unwired: 1 in, 6 out]
                                n864 = local read "MFLI-1-Settings"() -> (w997:T1)
                                n865 = Unbundle By Name(w997) -> ("Aux Out 3 Scale"=w996:dbl)
                                n866 = call-poly "ziSetValue.vi"("Value"=w996, "Path"="auxouts/3/scale", "Handle In"=w999) -> ("Handle Out"=w998:T4)  [unwired: 2 in, 1 out]
                              }
                              event Value Change {
                                n867 = event-data() -> ()  [unwired: 1 in, 6 out]
                                n868 = local read "MFLI-1-Settings"() -> (w1002:T1)
                                n869 = Unbundle By Name(w1002) -> ("Aux Out 0 Offset"=w1001:dbl)
                                n870 = call-poly "ziSetValue.vi"("Value"=w1001, "Path"="auxouts/0/offset", "Handle In"=w1004) -> ("Handle Out"=w1003:T4)  [unwired: 2 in, 1 out]
                              }
                              event Value Change {
                                n871 = event-data() -> ()  [unwired: 1 in, 6 out]
                                n872 = local read "MFLI-1-Settings"() -> (w1007:T1)
                                n873 = Unbundle By Name(w1007) -> ("Aux Out 1 Offset"=w1006:dbl)
                                n874 = call-poly "ziSetValue.vi"("Value"=w1006, "Path"="auxouts/1/offset", "Handle In"=w1009) -> ("Handle Out"=w1008:T4)  [unwired: 2 in, 1 out]
                              }
                              event Value Change {
                                n875 = event-data() -> ()  [unwired: 1 in, 6 out]
                                n876 = local read "MFLI-1-Settings"() -> (w1012:T1)
                                n877 = Unbundle By Name(w1012) -> ("Aux Out 2 Offset"=w1011:dbl)
                                n878 = call-poly "ziSetValue.vi"("Value"=w1011, "Path"="auxouts/2/offset", "Handle In"=w1014) -> ("Handle Out"=w1013:T4)  [unwired: 2 in, 1 out]
                              }
                              event Value Change {
                                n879 = event-data() -> ()  [unwired: 1 in, 6 out]
                                n880 = local read "MFLI-1-Settings"() -> (w1017:T1)
                                n881 = Unbundle By Name(w1017) -> ("Aux Out 3 Offset"=w1016:dbl)
                                n882 = call-poly "ziSetValue.vi"("Value"=w1016, "Path"="auxouts/3/offset", "Handle In"=w1019) -> ("Handle Out"=w1018:T4)  [unwired: 2 in, 1 out]
                              }
                            }
                          }
                          frame #2 {
                            n883 = global write "Instrument_Setup.vi" "Update Lockins"(FALSE) -> ()
                          }
                        }
                      }
                    }
                  }
                  frame #1 {
                    n884 = flat-sequence {
                      frame #0 {
                        n885 = local read "Lock-in Reference"() -> (w1023:u16)
                        n886 = local read "MFLI-1-Settings"() -> (w1024:T1)
                        n887 = case shown="0, Default" w1023 {
                          tunnel: w1024 -> [w1025 w1026 w1027]
                          frame 0, Default {
                            n888 = global write "Instrument_Setup.vi" "MFLI-1-Settings"(w1025) -> ()
                          }
                          frame 1 {
                            n889 = global write "Instrument_Setup.vi" "MFLI-1-Settings"(w1026) -> ()
                          }
                          frame 2 {
                            n890 = global write "Instrument_Setup.vi" "MFLI-1-Settings"(w1027) -> ()
                          }
                        }
                      }
                      frame #1 {
                        n891 = global read "Instrument_Setup.vi" "Update Lockins"() -> (w1030:bool)
                        n892 = And(x=w1030, y=TRUE) -> (x .and. y?=w1028:bool)
                        n893 = case shown="False" w1028 {
                          frame False {
                          }
                          frame True {
                            n894 = global write "Instrument_Setup.vi" "Update Lockins"(FALSE) -> ()
                          }
                        }
                      }
                    }
                  }
                  frame #2 {
                    n895 = Unbundle By Name(w1036) -> ("Demod 3 Zero Phase"=w1032:bool, "Demod 2 Zero Phase"=w1033:bool, "Demod 1 Zero Phase"=w1034:bool, "Demod 0 Zero Phase"=w1035:bool)
                    n896 = case shown="True" w1035 {
                      tunnel: w1041 -> [w1057 w1059]
                      tunnel: [w1057 w1058] -> w1040
                      frame False {
                      }
                      frame True {
                        n897 = call-poly "ziSetValue.vi"("Value"=1.0 ("Value In"), "Path"="demods/0/phaseadjust", "Handle In"=w1059) -> ("Handle Out"=w1058:T4)  [unwired: 2 in, 1 out]
                      }
                    }
                    n898 = case shown="True" w1034 {
                      tunnel: w1040 -> [w1052 w1054]
                      tunnel: [w1052 w1053] -> w1039
                      frame False {
                      }
                      frame True {
                        n899 = call-poly "ziSetValue.vi"("Value"=1.0 ("Value In"), "Path"="demods/1/phaseadjust", "Handle In"=w1054) -> ("Handle Out"=w1053:T4)  [unwired: 2 in, 1 out]
                      }
                    }
                    n900 = case shown="True" w1033 {
                      tunnel: w1039 -> [w1047 w1049]
                      tunnel: [w1047 w1048] -> w1038
                      frame False {
                      }
                      frame True {
                        n901 = call-poly "ziSetValue.vi"("Value"=1.0 ("Value In"), "Path"="demods/2/phaseadjust", "Handle In"=w1049) -> ("Handle Out"=w1048:T4)  [unwired: 2 in, 1 out]
                      }
                    }
                    n902 = case shown="True" w1032 {
                      tunnel: w1038 -> [w1042 w1044]
                      tunnel: [w1042 w1043] -> w1037
                      frame False {
                      }
                      frame True {
                        n903 = call-poly "ziSetValue.vi"("Value"=1.0 ("Value In"), "Path"="demods/3/phaseadjust", "Handle In"=w1044) -> ("Handle Out"=w1043:T4)  [unwired: 2 in, 1 out]
                      }
                    }
                  }
                  frame #3 {
                    n904 = Unbundle By Name(w1063) -> ("Update Osci"=w1062:bool)
                    n905 = case shown="True" w1062 {
                      tunnel: w1065 -> [w1066 w1073]
                      tunnel: w1063 -> [_ w1071]
                      tunnel: [w1066 w1067] -> w1064
                      frame False {
                      }
                      frame True {
                        n906 = local read "MFL_Monitor"() -> (w1077:T2)
                        n907 = Unbundle By Name(w1071) -> ("Range (V)"=w1074:dbl)
                        n908 = Unbundle By Name(w1071) -> ("Offset (V)"=w1068:dbl)
                        n909 = Unbundle By Name(w1077) -> ("Range (V)"=w1075:dbl, "Offset (V)"=w1070:dbl)
                        n910 = Not Equal?(x=w1074, y=w1075) -> (x != y?=w1076:bool)
                        n911 = case shown="True" w1076 {
                          tunnel: w1074 -> [_ w1086]
                          tunnel: w1073 -> [w1083 w1085]
                          tunnel: [w1083 w1084] -> w1072
                          frame False {
                          }
                          frame True {
                            n912 = call-poly "ziSetValue.vi"("Value"=w1086, "Path"="sigouts/0/range", "Handle In"=w1085) -> ("Handle Out"=w1084:T4)  [unwired: 2 in, 1 out]
                          }
                        }
                        n913 = Not Equal?(x=w1070, y=w1068) -> (x != y?=w1069:bool)
                        n914 = case shown="True" w1069 {
                          tunnel: w1072 -> [w1078 w1081]
                          tunnel: [w1078 w1080] -> w1067
                          tunnel: w1068 -> [_ w1079]
                          frame False {
                          }
                          frame True {
                            n915 = call-poly "ziSetValue.vi"("Value"=w1079, "Path"="sigouts/0/offset", "Handle In"=w1081) -> ("Handle Out"=w1080:T4)  [unwired: 2 in, 1 out]
                          }
                        }
                      }
                    }
                  }
                  frame #4 {
                    n916 = Unbundle By Name(w1089) -> ("Update Osci"=w1088:bool)
                    n917 = case shown="True" w1088 {
                      tunnel: w1089 -> [_ w1111]
                      tunnel: w1091 -> [w1092 w1107]
                      tunnel: [w1092 w1093] -> w1090
                      frame False {
                      }
                      frame True {
                        n918 = local read "MFL_Monitor"() -> (w1110:T2)
                        n919 = Unbundle By Name(w1110) -> ("Osc 0 Freq"=w1108:dbl, "Osc 1 Freq"=w1103:dbl, "Osc 2 Freq"=w1101:dbl, "Osc 3 Freq"=w1097:dbl)
                        n920 = Unbundle By Name(w1111) -> ("Osc 0 Freq"=w1106:dbl, "Osc 1 Freq"=w1102:dbl, "Osc 2 Freq"=w1099:dbl, "Osc 3 Freq"=w1095:dbl)
                        n921 = Not Equal?(x=w1106, y=w1108) -> (x != y?=w1109:bool)
                        n922 = case shown="True" w1109 {
                          tunnel: w1107 -> [w1127 w1130]
                          tunnel: w1106 -> [_ w1129]
                          tunnel: [w1127 w1128] -> w1105
                          frame False {
                          }
                          frame True {
                            n923 = call-poly "ziSetValue.vi"("Value"=w1129, "Path"="oscs/0/freq", "Handle In"=w1130) -> ("Handle Out"=w1128:T4)  [unwired: 2 in, 1 out]
                          }
                        }
                        n924 = Not Equal?(x=w1102, y=w1103) -> (x != y?=w1104:bool)
                        n925 = Not Equal?(x=w1099, y=w1101) -> (x != y?=w1100:bool)
                        n926 = Not Equal?(x=w1095, y=w1097) -> (x != y?=w1096:bool)
                        n927 = case shown="True" w1104 {
                          tunnel: w1105 -> [w1122 w1124]
                          tunnel: [w1122 w1125] -> w1098
                          tunnel: w1102 -> [_ w1123]
                          frame False {
                          }
                          frame True {
                            n928 = call-poly "ziSetValue.vi"("Value"=w1123, "Path"="oscs/1/freq", "Handle In"=w1124) -> ("Handle Out"=w1125:T4)  [unwired: 2 in, 1 out]
                          }
                        }
                        n929 = case shown="True" w1100 {
                          tunnel: w1099 -> [_ w1120]
                          tunnel: w1098 -> [w1117 w1119]
                          tunnel: [w1117 w1118] -> w1094
                          frame False {
                          }
                          frame True {
                            n930 = call-poly "ziSetValue.vi"("Value"=w1120, "Path"="oscs/2/freq", "Handle In"=w1119) -> ("Handle Out"=w1118:T4)  [unwired: 2 in, 1 out]
                          }
                        }
                        n931 = case shown="True" w1096 {
                          tunnel: w1095 -> [_ w1113]
                          tunnel: w1094 -> [w1112 w1115]
                          tunnel: [w1112 w1114] -> w1093
                          frame False {
                          }
                          frame True {
                            n932 = call-poly "ziSetValue.vi"("Value"=w1113, "Path"="oscs/2/freq", "Handle In"=w1115) -> ("Handle Out"=w1114:T4)  [unwired: 2 in, 1 out]
                          }
                        }
                      }
                    }
                  }
                  frame #5 {
                    n933 = local read "MFL_Monitor"() -> (w1149:T2)
                    n934 = Unbundle By Name(w1149) -> ("Ampl 0"=w1148:dbl, "Ampl 1"=w1144:dbl, "Ampl 2"=w1140:dbl, "Ampl 3"=w1135:dbl)
                    n935 = Unbundle By Name(w1150) -> ("Ampl 0"=w1145:dbl, "Ampl 1"=w1141:dbl, "Ampl 2"=w1137:dbl, "Ampl 3"=w1134:dbl)
                    n936 = Not Equal?(x=w1145, y=w1148) -> (x != y?=w1147:bool)
                    n937 = Not Equal?(x=w1141, y=w1144) -> (x != y?=w1143:bool)
                    n938 = Not Equal?(x=w1137, y=w1140) -> (x != y?=w1139:bool)
                    n939 = Not Equal?(x=w1134, y=w1135) -> (x != y?=w1133:bool)
                    n940 = case shown="True" w1147 {
                      tunnel: w1146 -> [w1166 w1169]
                      tunnel: [w1166 w1168] -> w1142
                      tunnel: w1145 -> [_ w1167]
                      frame False {
                      }
                      frame True {
                        n941 = call-poly "ziSetValue.vi"("Value"=w1167, "Path"="sigouts/0/amplitudes/0", "Handle In"=w1169) -> ("Handle Out"=w1168:T4)  [unwired: 2 in, 1 out]
                      }
                    }
                    n942 = case shown="True" w1143 {
                      tunnel: w1142 -> [w1161 w1164]
                      tunnel: [w1161 w1163] -> w1138
                      tunnel: w1141 -> [_ w1162]
                      frame False {
                      }
                      frame True {
                        n943 = call-poly "ziSetValue.vi"("Value"=w1162, "Path"="sigouts/0/amplitudes/1", "Handle In"=w1164) -> ("Handle Out"=w1163:T4)  [unwired: 2 in, 1 out]
                      }
                    }
                    n944 = case shown="True" w1139 {
                      tunnel: w1138 -> [w1156 w1159]
                      tunnel: [w1156 w1158] -> w1136
                      tunnel: w1137 -> [_ w1157]
                      frame False {
                      }
                      frame True {
                        n945 = call-poly "ziSetValue.vi"("Value"=w1157, "Path"="sigouts/0/amplitudes/2", "Handle In"=w1159) -> ("Handle Out"=w1158:T4)  [unwired: 2 in, 1 out]
                      }
                    }
                    n946 = case shown="True" w1133 {
                      tunnel: w1136 -> [w1151 w1154]
                      tunnel: w1134 -> [_ w1153]
                      tunnel: [w1151 w1152] -> w1132
                      frame False {
                      }
                      frame True {
                        n947 = call-poly "ziSetValue.vi"("Value"=w1153, "Path"="sigouts/0/amplitudes/3", "Handle In"=w1154) -> ("Handle Out"=w1152:T4)  [unwired: 2 in, 1 out]
                      }
                    }
                  }
                }
              }
            }
          }
          frame #4 {
            n948 = local read "Lock-in Reference"() -> (w1171:u16)
            n949 = global read "Instrument_Setup.vi" "Set-Lockin-Sens"() -> (w1174:u16)
            n950 = case shown="0, Default" w1174 {
              tunnel: w1173 -> [w1182 w1200 w1209]
              tunnel: [w1180 w1199 w1208] -> w1172
              tunnel: w1171 -> [w1183 _ _]
              frame 0, Default {
                n951 = local read "MFL_Monitor"() -> (w1177:T2)
                n952 = Unbundle By Name(w1177) -> ("Auto-Range"=w1176:bool)
                n953 = global read "Data_Display_global.vi" "Lock-In-Sensitivity-Cluster"() -> (w1184:T8)
                n954 = case shown="0, Default" w1183 {
                  tunnel: [w1191 w1194 w1195] -> w1178
                  tunnel: w1184 -> [w1192 w1193 w1196]
                  frame 0, Default {
                    n955 = Unbundle By Name(w1192) -> ("Sensitivity Setpoint 1"=w1191:i32)
                  }
                  frame 1 {
                    n956 = Unbundle By Name(w1193) -> ("Sensitivity Setpoint 2"=w1194:i32)
                  }
                  frame 2 {
                    n957 = Unbundle By Name(w1196) -> ("Sensitivity Setpoint 3"=w1195:i32)
                  }
                }
                n958 = case shown="True" w1176 {
                  tunnel: w1182 -> [w1186 w1189]
                  tunnel: [w1186 w1188] -> w1181
                  frame False {
                  }
                  frame True {
                    n959 = call-poly "ziSetValue.vi"("Value"=0, "Path"="sigouts/0/autorange", "Handle In"=w1189) -> ("Handle Out"=w1188:T4)  [unwired: 2 in, 1 out]
                  }
                }
                n960 = local read "MFLI-1-Settings"() -> (w1179:T1)
                n961 = Bundle By Name(cluster=w1179, "Range (V)"=w1178) -> (w1175:T1)
                n962 = global write "Instrument_Setup.vi" "MFLI-1-Settings"(w1175) -> ()
                n963 = local write "MFLI-1-Settings"(w1175) -> ()
                n964 = call-poly "ziSetValue.vi"("Value"=w1178, "Path"="sigouts/0/range", "Handle In"=w1181) -> ("Handle Out"=w1180:T4)  [unwired: 2 in, 1 out]
              }
              frame 1 {
                n965 = local read "MFL_Monitor"() -> (w1198:T2)
                n966 = Unbundle By Name(w1198) -> ("Auto-Range"=w1197:bool)
                n967 = case shown="False" w1197 {
                  tunnel: w1200 -> [w1202 w1205]
                  tunnel: [w1201 w1205] -> w1199
                  frame False {
                    n968 = call-poly "ziSetValue.vi"("Value"=1, "Path"="sigouts/0/autorange", "Handle In"=w1202) -> ("Handle Out"=w1201:T4)  [unwired: 2 in, 1 out]
                  }
                  frame True {
                  }
                }
              }
              frame 2 {
                n969 = local read "MFL_Monitor"() -> (w1207:T2)
                n970 = Unbundle By Name(w1207) -> ("Auto-Range"=w1206:bool)
                n971 = case shown="False" w1206 {
                  tunnel: w1209 -> [w1210 w1212]
                  tunnel: [w1210 w1211] -> w1208
                  frame False {
                  }
                  frame True {
                    n972 = call-poly "ziSetValue.vi"("Value"=0, "Path"="sigouts/0/autorange", "Handle In"=w1212) -> ("Handle Out"=w1211:T4)  [unwired: 2 in, 1 out]
                  }
                }
              }
            }
          }
          frame #5 {
            n973 = local read "Lock-in Reference"() -> (w1216:u16)
            n974 = local read "MFL_Monitor"() -> (w1215:T2)
            n975 = case shown="2" w1216 {
              tunnel: w1215 -> [w1218 w1222 w1229]
              frame 0, Default {
                n976 = global read "Data_Display_global.vi" "Lock-In-Running-Cluster"() -> (w1221:T9)
                n977 = Bundle By Name(cluster=w1221, "zurich_Lock_in-running"=TRUE) -> (w1219:T9)
                n978 = global write "Data_Display_global.vi" "Lock-In-Running-Cluster"(w1219) -> ()
                n979 = global write "Data_Display_global.vi" "MFL_Monitor"(w1218) -> ()
              }
              frame 1 {
                n980 = global read "Data_Display_global.vi" "Lock-In-Running-Cluster"() -> (w1225:T9)
                n981 = Bundle By Name(cluster=w1225, "zurich_Lock_in-running"=TRUE) -> (w1223:T9)
                n982 = global write "Data_Display_global.vi" "Lock-In-Running-Cluster"(w1223) -> ()
                n983 = global write "Data_Display_global.vi" "MFL_Monitor"(w1222) -> ()
              }
              frame 2 {
                n984 = global read "Data_Display_global.vi" "Lock-In-Running-Cluster"() -> (w1228:T9)
                n985 = Bundle By Name(cluster=w1228, "zurich_Lock_in-running"=TRUE) -> (w1226:T9)
                n986 = global write "Data_Display_global.vi" "Lock-In-Running-Cluster"(w1226) -> ()
                n987 = global write "Data_Display_global.vi" "MFL_Monitor"(w1229) -> ()
              }
            }
          }
          frame #6 {
            n988 = local read "Lock-in Reference"() -> (w1231:u16)
            n989 = case shown="True" "Stop" {
              tunnel: w1231 -> [_ w1233]
              frame False {
              }
              frame True {
                n990 = case shown="2" w1233 {
                  frame 0, Default {
                    n991 = global read "Data_Display_global.vi" "Lock-In-Running-Cluster"() -> (w1236:T9)
                    n992 = Bundle By Name(cluster=w1236, "zurich_Lock_in-running"=FALSE) -> (w1234:T9)
                    n993 = global write "Data_Display_global.vi" "Lock-In-Running-Cluster"(w1234) -> ()
                  }
                  frame 1 {
                    n994 = global read "Data_Display_global.vi" "Lock-In-Running-Cluster"() -> (w1239:T9)
                    n995 = Bundle By Name(cluster=w1239, "zurich_Lock_in-running"=FALSE) -> (w1237:T9)
                    n996 = global write "Data_Display_global.vi" "Lock-In-Running-Cluster"(w1237) -> ()
                  }
                  frame 2 {
                    n997 = global read "Data_Display_global.vi" "Lock-In-Running-Cluster"() -> (w1242:T9)
                    n998 = Bundle By Name(cluster=w1242, "zurich_Lock_in-running"=FALSE) -> (w1240:T9)
                    n999 = global write "Data_Display_global.vi" "Lock-In-Running-Cluster"(w1240) -> ()
                  }
                }
              }
            }
          }
        }
      }
    }
    frame #4 {
      n1000 = local read "MFL_Monitor"() -> (w1245:T2)
      n1001 = Bundle By Name(cluster=w1245, "Connected ?"=FALSE) -> (w1244:T2)
      n1002 = local write "MFL_Monitor"(w1244) -> ()
    }
  }
  n1003 = call "ziClose.vi"("Handle In"=w8) -> ()  [unwired: 3 in, 2 out]
